vi "Process.vi"(8 "error in":errorcluster, 11 "Instrument.Lockin":refnum<class "Instrument.Lockin.lvclass">) -> (0 "error out":errorcluster, 3 "Instrument.Lockin out":refnum<class "Instrument.Lockin.lvclass">)   [LabVIEW 2019, in "Instrument.Lockin.lvlib" / "Instrument.Lockin.lvclass"]
doc: "---------------------------------------------------------------\nJKI State Machine Objects™\nhttp://jki.net/state-machine-objects/\nCopyright (C) 2005-2015, JKI <info@jki.net>\nALL RIGHTS RESERVED"
uses:
  Instrument.Lockin.lvclass
  C:/Program Files/National Instruments/LabVIEW 2019/vi.lib/JKI/JKI SMO/SMO/SMO.lvclass
  C:/Program Files/National Instruments/LabVIEW 2019/user.lib/LevyLab/Instrument Framework/Instrument/Instrument.lvclass
  Typedefs/API/Lockin.Commands.Local--Enum.ctl
  Instrument.Lockin.lvclass/Instrument.Lockin.ctl
  Typedefs/Lockin.Logging Mode--Enum.ctl
  Instrument.DAQ/Typedefs/PublicEvents--DAQ.getSweepWaveforms.ctl
  <vilib>/JKI/JKI SMO/SMO/SMO.lvclass/SMO.ctl
  Instrument.DAQ/Typedefs/Status--enum.ctl
  26abb908-d0dd-4bb2-b0ae-9417a76ac08a.vi
  58bdca10-aee7-4643-9696-ab134e43fedf.vi
  370a30f5-6ed9-43ab-971d-2debb7bc2492.vi
  5bf8e0f0-076c-483f-9499-ed5c5f42f10f.vi
  57cf7fb7-944b-4fe2-b1a2-0684563889c1.vi
  f640c324-6c77-497d-a9f4-fdf294fa3808.vi
  2ccda5d8-d2df-4877-8897-cb36dbf858a1.vi
  7ebf71aa-15a6-4da8-8ab8-2681a3011f9e.vi
  cf0dbf68-f98d-44ab-94b5-1d1e0573f492.vi
  befd05cc-8908-477d-a2f5-b8fbe5183ab0.vi
  4dcf9d6e-caf6-43ae-ab2a-813b64901b82.vi
  0479806f-3f82-4f4d-965e-31251a6a8c57.vi
  682026ae-b6e8-4d7d-90ad-286834dc1f4b.vi
  2a868a51-49ac-40d0-a5d8-0cf59a96bd77.vi
  26abb908-d0dd-4bb2-b0ae-9417a76ac08a.vi/314341ff-f36a-4754-8de1-4f8aeb5d3876.vi
  26abb908-d0dd-4bb2-b0ae-9417a76ac08a.vi/d069243e-0f6a-4917-95a4-9b44f4392aec.vi
  58bdca10-aee7-4643-9696-ab134e43fedf.vi/f87b1427-1328-4423-a40d-becc2975277f.vi
  58bdca10-aee7-4643-9696-ab134e43fedf.vi/ed747cf9-ba41-4379-ab59-768bb8ae5ff5.vi
  57cf7fb7-944b-4fe2-b1a2-0684563889c1.vi/1fd4b456-2f60-4d06-9716-df1c45004a86.vi
  57cf7fb7-944b-4fe2-b1a2-0684563889c1.vi/c11c9ad7-4649-4a85-b536-b866ca836ca1.vi
  f640c324-6c77-497d-a9f4-fdf294fa3808.vi/dbd296fc-8f34-43a8-ad34-5f6fb66ed20d.vi
  f640c324-6c77-497d-a9f4-fdf294fa3808.vi/6db23667-e41e-42f6-b96f-5bc501eef0b9.vi
  2ccda5d8-d2df-4877-8897-cb36dbf858a1.vi/344e3d59-91b1-4f61-87d6-f8dd4cdbc25b.vi
  2ccda5d8-d2df-4877-8897-cb36dbf858a1.vi/d2d6577b-fb43-4e7b-ace1-03f46b56d867.vi
  7ebf71aa-15a6-4da8-8ab8-2681a3011f9e.vi/60f027cd-f7ba-4b68-b22c-bc105befc801.vi
  7ebf71aa-15a6-4da8-8ab8-2681a3011f9e.vi/6c60f1e5-9ce0-4de3-ba4a-93b0668e9427.vi
  befd05cc-8908-477d-a2f5-b8fbe5183ab0.vi/b24fcc70-6624-4032-8476-943c5eb956bf.vi
  befd05cc-8908-477d-a2f5-b8fbe5183ab0.vi/cde51830-ddf3-45a8-9955-a1d629d46cfc.vi
  4dcf9d6e-caf6-43ae-ab2a-813b64901b82.vi/85e7a3df-5796-4879-b3a1-48313e8334c0.vi
  4dcf9d6e-caf6-43ae-ab2a-813b64901b82.vi/8e8c5bfe-5699-4deb-abb3-b8b413165a55.vi
  0479806f-3f82-4f4d-965e-31251a6a8c57.vi/af1f2937-4b31-4fa9-86ad-f8d3a4898bc2.vi
  0479806f-3f82-4f4d-965e-31251a6a8c57.vi/3be0beb5-3802-4edd-aa59-089ac39f706e.vi
  <vilib>/dlg_ctls.llb/Space Constant.vi
  <vilib>/AdvancedString/1D String Array to Delimited String.vi
  <vilib>/JKI/JKI SMO/SMO/Private/ReftoDVR--SMO.vi
  <vilib>/Utility/Data Type/Get Type Information.vi
  <vilib>/Utility/Data Type/Get Numeric Information.vi
  <userlib>/_OpenG.lib/lvdata/lvdata.llb/Unwrap VVariant__ogtk.vi
  <vilib>/JDP Science/JSONtext/Variant to JSON Text.vi
  <userlib>/LevyLab/Instrument Framework/Instrument/API/Instrument.sendMessageToProcess (string).vi
  <vilib>/JDP Science/JSONtext/LVClass Serializer/JSONtext LVClass Serializer.lvclass
  <vilib>/JKI/JKI SMO/SMO/SMO.lvclass
  <userlib>/LevyLab/Instrument Framework/Instrument Types/Lockin/Instrument.LockinAPI.lvclass
  <userlib>/LevyLab/Debug/Debug.lvlib
  Instrument.DAQ/Instrument.DAQ.lvclass
  <userlib>/LevyLab/Instrument Framework/Instrument/Instrument.lvclass
panel:
  in  "LOG":bool
  out "String":string
  # "Multichannel Lockin"
  # "For instructions on how to use the JKI State Machine Objects, examples and video tutorials, visit:\nhttp://jki.net/state-machine-objects/\n\nJKI State Machine Objects™\nhttp://jki.net/state-machine-objects/\nCopyright (C) 2005-2015, JKI <info@jki.net>\nALL RIGHTS RESERVED"
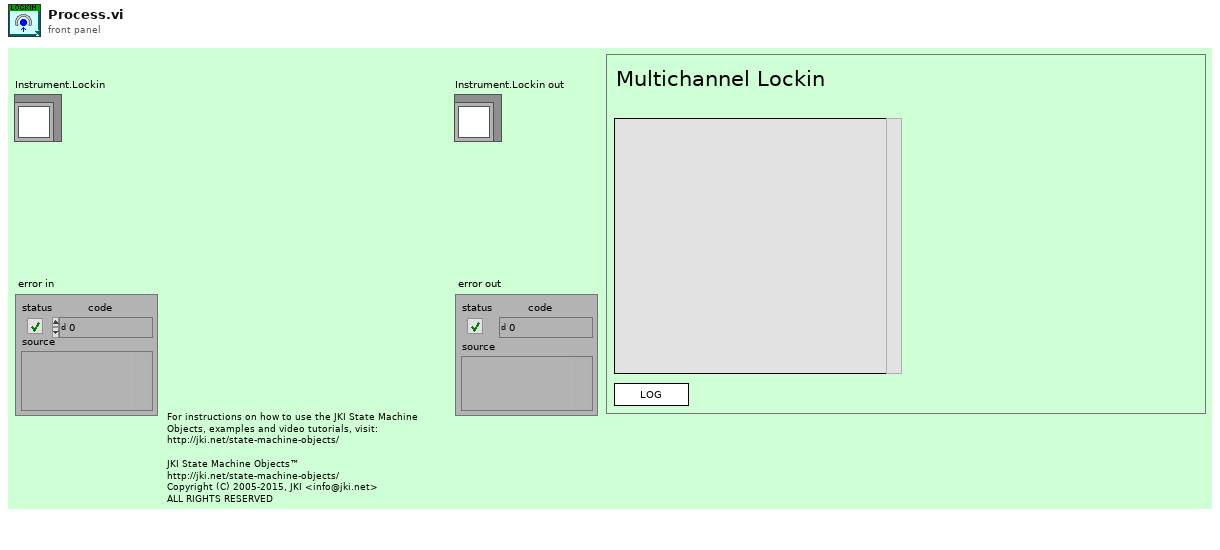
[diagram p1: front panel]
types:
  T1 = typedef "Instrument.Lockin.lvlib/Instrument.Lockin.lvclass/Lockin.Commands.Local--Enum.ctl" = enum16{"autoConfigureDAQ", "setSimulationMode", "zeroPhase", "setCalibration", "setPreFilter", "setFrequencyLink", "setAmplitudeLimit", "setDCLimit", "setDutyCycle", "setSamplingDecimationPreDSP", "setSamplingDecimationPostDSP", "setSamplingMode", "setSamplingFsMultiplier", "setSamplingFsOutput", "setSamplingRefreshRate", "setData_State", "setData_DAQ", "setData_Sampling", "setData_Waveforms", "setData_Results", "setData_SweepWaveforms", "setData_AIChannels", "setData_AOChannels", "setData_REFChannels", "setData_InputGain", "setData_OutputGain", "showUI", "setAI", "setOffset", "setOffsetMode"}
  T2 = typedef "Instrument.Lockin.lvlib/Instrument.Lockin.lvclass/Lockin.Logging Mode--Enum.ctl" = enum16{"enabled", "disabled"}
  T3 = enum32{"invalid app kind", "Development System", "Run Time System", "Student Edition", "Embedded LabVIEW", "Evaluation", "Custom"}
  T4 = enum32{"Invalid", "Standard", "Closed", "Hidden", "Minimized", "Maximized"}
  T5 = typedef "Instrument.Lockin.lvlib/Instrument.DAQ.lvclass/Status--enum.ctl" = enum16{"idle", "created", "started", "stopped", "sweeping"}
  T6 = typedef "Instrument.Lockin.lvlib/Instrument.DAQ.lvclass/PublicEvents--DAQ.getSweepWaveforms.ctl" = cluster{"AO":waveform(dbl)[], "AI":waveform(dbl)[], "X":waveform(dbl)[], "Y":waveform(dbl)[]}
  T7 = typedef "SMO.lvclass/SMOState --Enum.ctl" = enum16{"unknown", "Created", "Started", "Stopped"}
  T8 = cluster{"Core":cluster{"Current VI Reference":refnum<vi>, "Close Panel on Exit?":bool, "Last Error":cluster{"error":errorcluster, "previous state":string, "remaining states":string}, "Shutdown?":bool}, "SelfRef":refnum<class "Instrument.Lockin.lvclass">, "logConfiguration":bool, "SweepWaveformsBuffer":T6}
  T9 = typedef "Instrument.Lockin.lvlib/Instrument.DAQ.lvclass/DAQ.Configuration--Cluster--Array.ctl" = T10[]
  T10 = typedef "Instrument.Lockin.lvlib/Instrument.DAQ.lvclass/DAQ.Configuration--Cluster.ctl" = cluster{"Device":string, "Lockin.AO":string, "AO.Ch":string, "AO.Range":T11, "AO terminal config":T12, "Lockin.AI":string, "AI.Ch":string, "AI.Range":T13, "AI.Coupling":T14, "AI terminal config":T12}
  T11 = typedef "Instrument.Lockin.lvlib/Instrument.DAQ.lvclass/DAQ.Config.AO.Range--enum.ctl" = enum16{"±0.1", "±1.0", "±3.5", "±10.0", ""}
  T12 = typedef "Instrument.Lockin.lvlib/Instrument.DAQ.lvclass/DAQ.TerminalConfiguration--ring.ctl" = i32
  T13 = typedef "Instrument.Lockin.lvlib/Instrument.DAQ.lvclass/DAQ.Config.AI.Range--enum.ctl" = enum16{"±0.316", "±1.00", "±3.16", "±10.0", "±31.6", "±42.4", ""}
  T14 = typedef "Instrument.Lockin.lvlib/Instrument.DAQ.lvclass/DAQ.Config.AI.Coupling--enum.ctl" = u16
  T15 = typedef "Instrument.Lockin.lvlib/Instrument.DAQ.lvclass/DAQ.Config.AO--Cluster--Array.ctl" = cluster{"Channels":tag, "Range":T11, "terminal configuration":T12, "Type":T16}[]
  T16 = typedef "Instrument.Lockin.lvlib/Instrument.DAQ.lvclass/DAQ.Type--enum.ctl" = enum16{"None", "USB-4431", "PXI-446x"}
  T17 = typedef "Instrument.Lockin.lvlib/Instrument.DAQ.lvclass/DAQ.Config.AI--Cluster--Array.ctl" = cluster{"Channels":tag, "Coupling":T14, "Range":T13, "terminal configuration":T12, "Type":T16}[]
  T18 = typedef "Instrument.Lockin.lvlib/Instrument.DAQ.lvclass/DAQ.Sampling--Cluster.ctl" = cluster{"Sampling":T19, "sample mode":i32, "Fs Mode":T20, "Fs Multiplier":dbl, "Refresh Rate (Hz)":dbl, "Decimation.PreDSP":i32, "Decimation.PostDSP":i32, "Fs.Output":dbl}
  T19 = typedef "Instrument.Lockin.lvlib/Instrument.DAQ.lvclass/DAQ.Sampling.Sampling--Cluster.ctl" = cluster{"Fs":dbl, "#s":i32}
  T20 = typedef "Instrument.Lockin.lvlib/Instrument.DAQ.lvclass/DAQ.Sampling.Fs Mode--enum.ctl" = enum16{"Manual", "Auto Fs", "Max Fs"}
  T21 = typedef "Instrument.Lockin.lvlib/Instrument.DAQ.lvclass/AI.Channel--Cluster--Array.ctl" = T22[]
  T22 = typedef "Instrument.Lockin.lvlib/Instrument.DAQ.lvclass/AI.Channel--Cluster.ctl" = cluster{"Enable?":bool, "Channel":i32, "References":u16[], "reference index":i32}
  T23 = typedef "Instrument.Lockin.lvlib/Instrument.DAQ.lvclass/AO.Channel--Cluster--Array.ctl" = T24[]
  T24 = typedef "Instrument.Lockin.lvlib/Instrument.DAQ.lvclass/AO.Channel--Cluster.ctl" = cluster{"Enable?":bool, "Channel":i32, "Amplitude":dbl, "Offset":dbl, "Frequency":dbl, "Phase":dbl, "Function":T25, "Sweeping?":bool, "Limit AC":bool, "Limit DC?":bool, "Duty Cycle":bool}
  T25 = typedef "Instrument.Lockin.lvlib/Instrument.DAQ.lvclass/AO.Channel.Function--Enum.ctl" = enum16{"sine", "square", "triangle", "saw"}
  T26 = typedef "Instrument.Lockin.lvlib/Instrument.DAQ.lvclass/REF.Channel--Cluster--Array.ctl" = T27[]
  T27 = typedef "Instrument.Lockin.lvlib/Instrument.DAQ.lvclass/REF.Channel--Cluster.ctl" = cluster{"Enable?":bool, "Channel":i32, "Frequency":dbl, "Phase":dbl, "TC":dbl, "Roll-Off":i32}
  T28 = typedef "Instrument.Lockin.lvlib/Instrument.DAQ.lvclass/PublicEvents--DAQ.getWaveforms.ctl" = cluster{"AO":waveform(dbl)[], "AI":waveform(dbl)[], "REF_X":waveform(dbl)[], "REF_Y":waveform(dbl)[], "X":waveform(dbl)[], "Y":waveform(dbl)[]}
  T29 = typedef "Instrument.Lockin.lvlib/Instrument.DAQ.lvclass/Results--Cluster.ctl" = cluster{"Time Stamp":timestamp, "Results (Dictionary)":cluster{"key":string, "value":dbl[]}[]}
  T30 = typedef "Instrument.Lockin.lvlib/Instrument.DAQ.lvclass/DeviceInfo--Cluster.ctl" = cluster{"DeviceName":string, "DevIsSimulated":bool, "DeviceSerialNumber":string, "ProductType":string, "ProductCategory":i32, "ProductNumber":u32, "ChassisNumber":u32, "SlotNumber":u32, "ChassisName":string, "ChassisSerialNumber":string, "DevTemp":dbl, "SelfCal.LastDate/Time":string, "SelfCal.LastTemp":dbl, "calibration due?":bool}
  T31 = typedef "Instrument.Lockin.lvlib/Instrument.DAQ.lvclass/DAQ.Calibration--Cluster--Array.ctl" = T32[]
  T32 = typedef "Instrument.Lockin.lvlib/Instrument.DAQ.lvclass/DAQ.Calibration--Cluster.ctl" = cluster{"Active Device":string, "SelfCal.LastDate/Time":dbl, "SelfCal.LastTemp":dbl, "DevTemp":dbl, "calibration due?":bool}
  T33 = cluster{"Current VI Reference":refnum<vi>, "Close Panel on Exit?":bool, "Last Error":cluster{"error":errorcluster, "previous state":string, "remaining states":string}, "Shutdown?":bool}
  T34 = typedef "Debug.lvlib/Attribute.Debug.lvclass/DebugBehavior.ctl" = enum16{"Normal", "Debug"}
  T35 = typedef "SMO.lvclass/Protected Events.ctl" = cluster{"StopProcesses":refnum<user-event>, "AbortProcesses":refnum<user-event>, "Config Changed":refnum<user-event>, "Dependency":refnum<user-event>}
  T36 = typedef "SMO.lvclass/Public Events.ctl" = cluster{"Error":refnum<user-event>, "State":refnum<user-event>, "Reserve State":refnum<user-event>}
  T37 = typedef "Instrument.Lockin.lvlib/Instrument.DAQ.lvclass/PublicEvents--Cluster.ctl" = cluster{"getAIChannels":refnum<user-event>, "getAOChannels":refnum<user-event>, "getREFChannels":refnum<user-event>, "getWaveforms":refnum<user-event>, "getResults":refnum<user-event>, "getSweepWaveforms":refnum<user-event>, "getCalibration":refnum<user-event>, "getDAQState":refnum<user-event>, "getDAQconfig":refnum<user-event>, "getInputGain":refnum<user-event>, "getOutputGain":refnum<user-event>, "getInputOffset":refnum<user-event>, "getSampling":refnum<user-event>, "getSweepChannels":refnum<user-event>, "getDeviceIDN":refnum<user-event>}
  T38 = typedef "Instrument.Lockin.lvlib/Instrument.Lockin.lvclass/PrivateEvents--Cluster.ctl" = cluster{"LogInterval":refnum<user-event>, "LogConfiguration":refnum<user-event>}
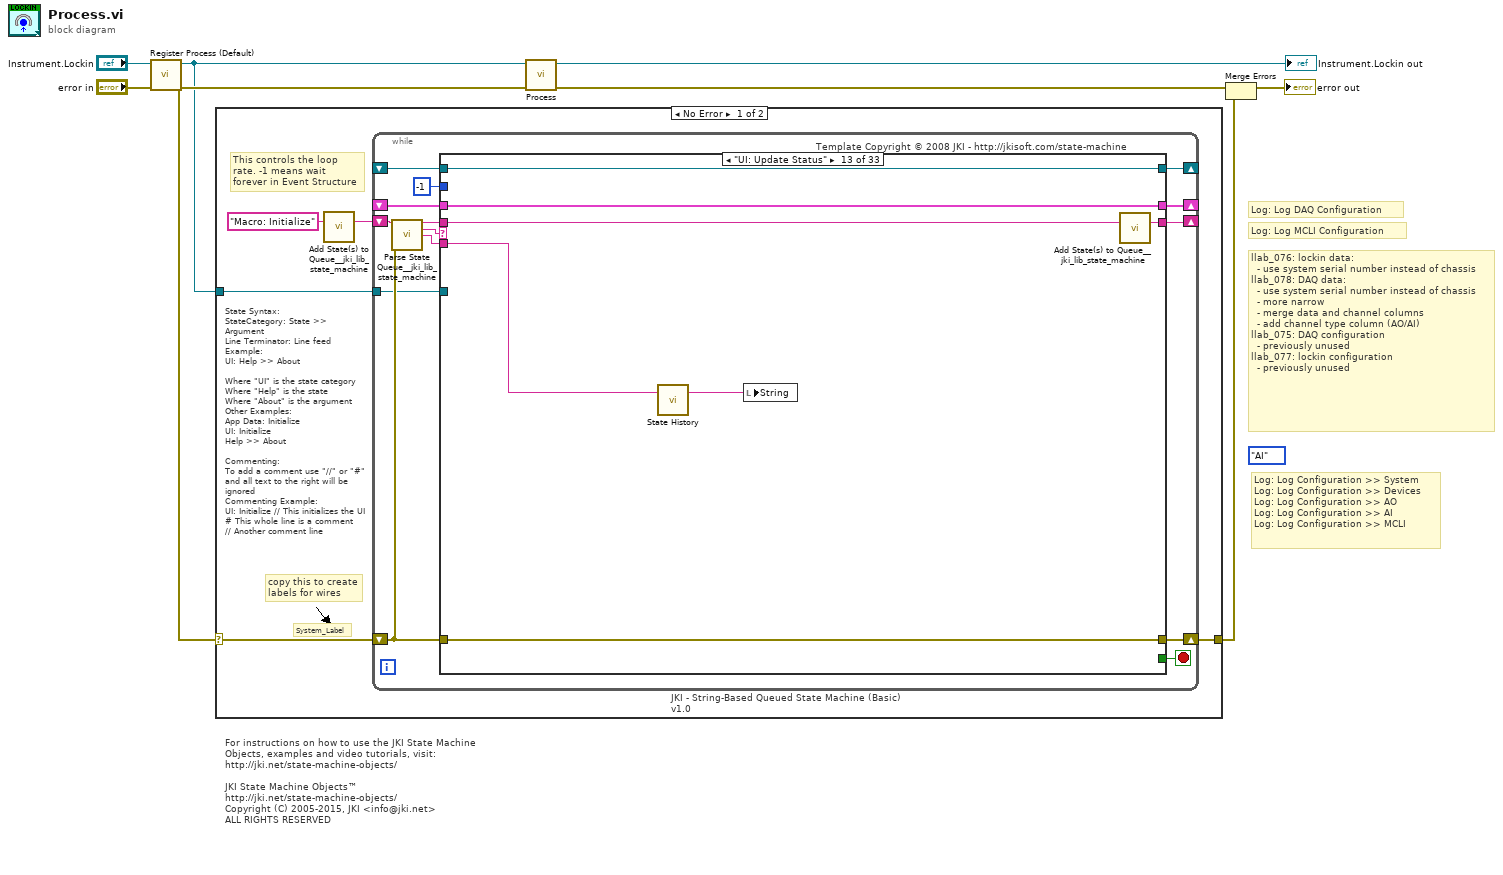
[diagram p0: block diagram]
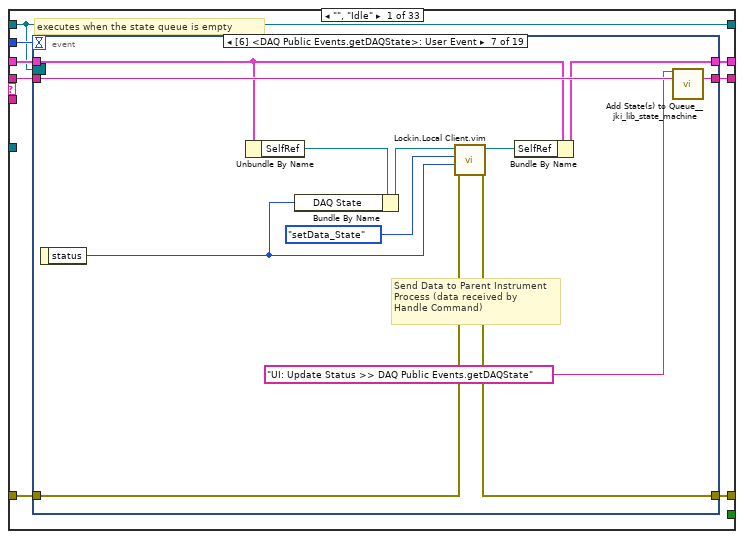
[diagram p2: hidden frame]
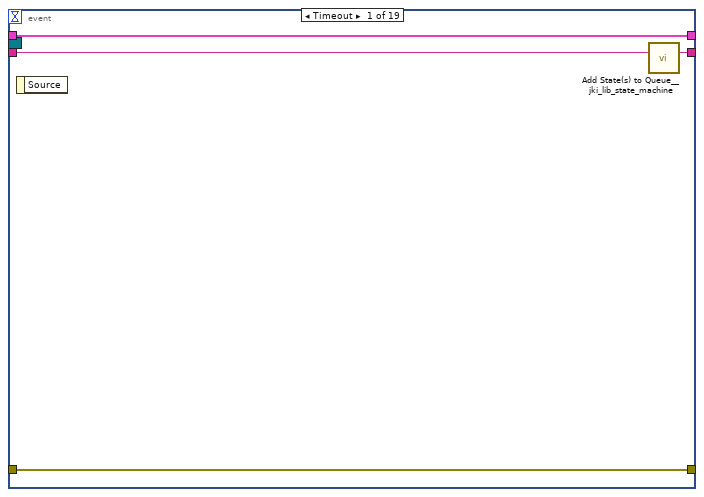
[diagram p3: hidden frame]
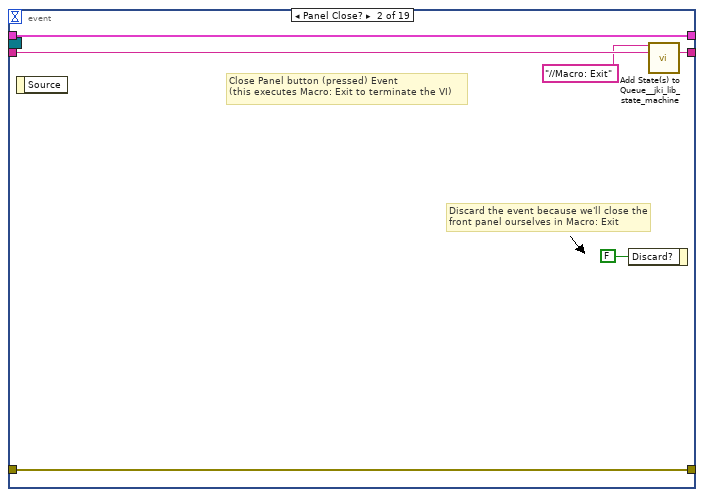
[diagram p4: hidden frame]
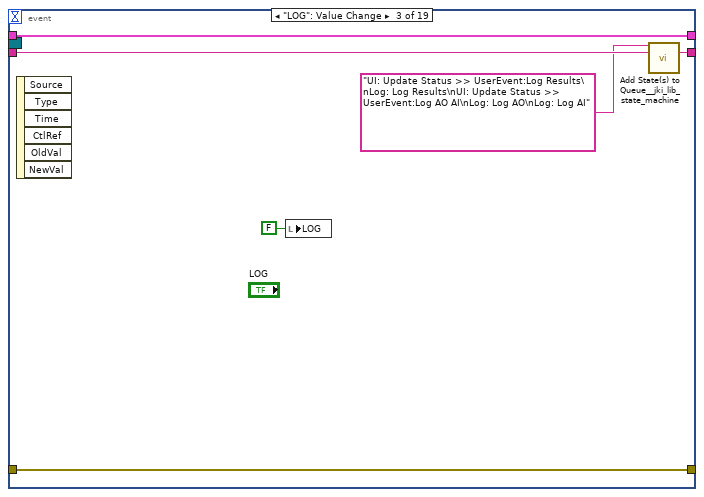
[diagram p5: hidden frame]
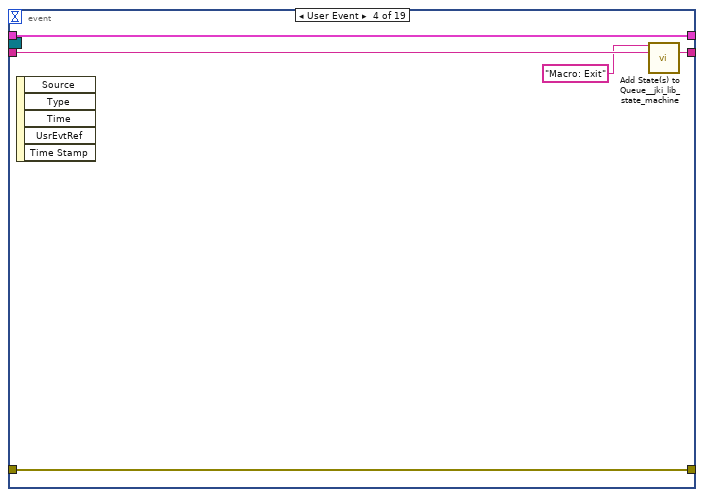
[diagram p6: hidden frame]
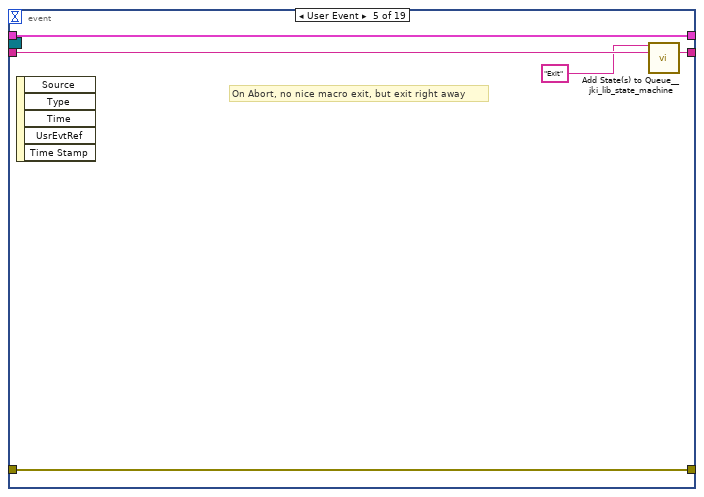
[diagram p7: hidden frame]
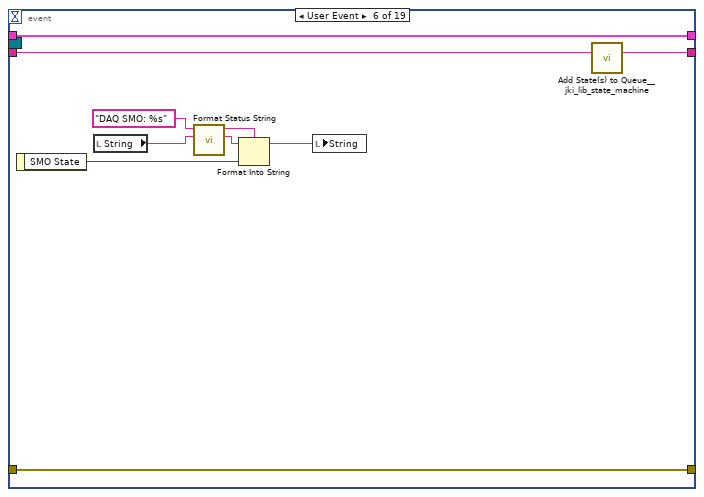
[diagram p8: hidden frame]
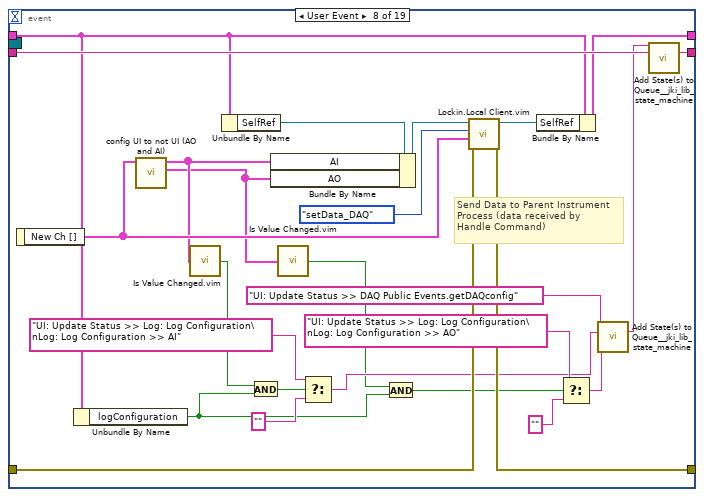
[diagram p9: hidden frame]
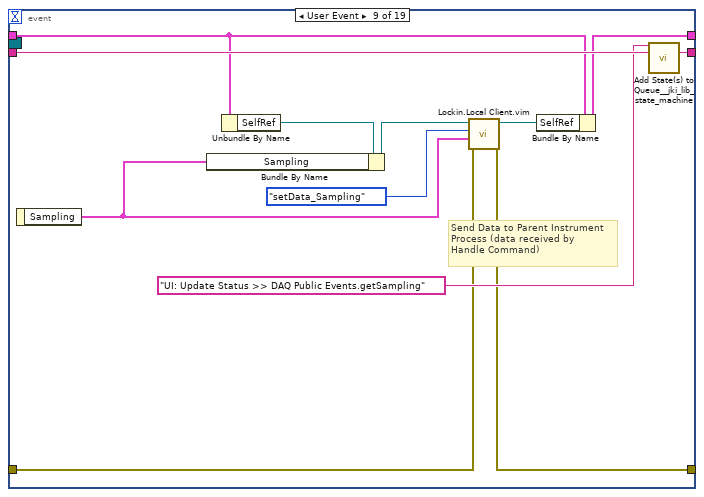
[diagram p10: hidden frame]
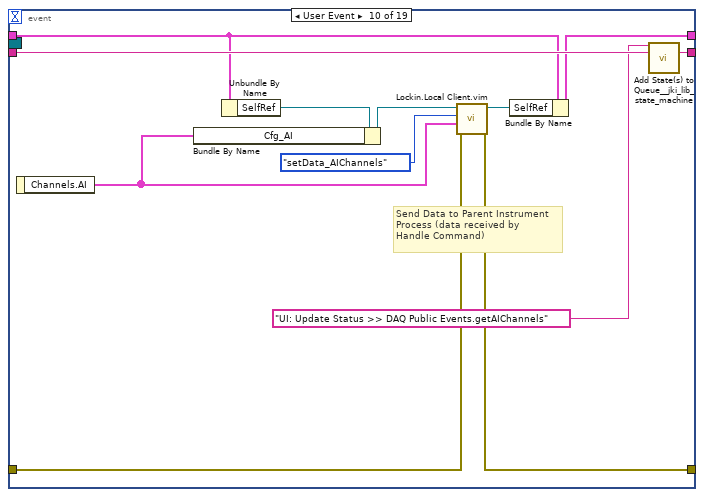
[diagram p11: hidden frame]
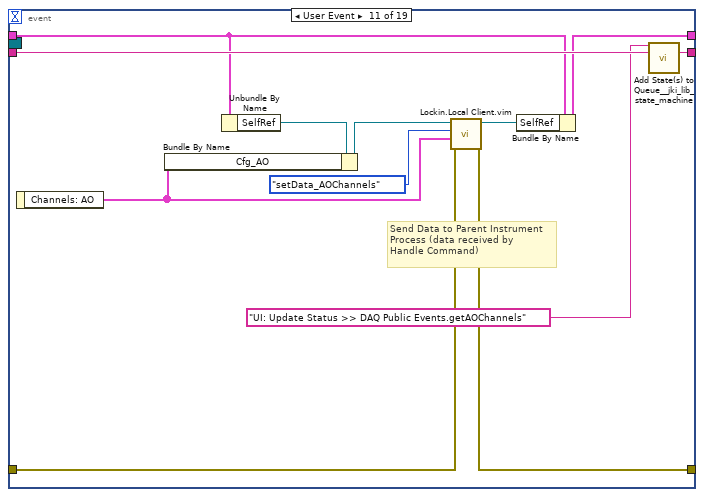
[diagram p12: hidden frame]
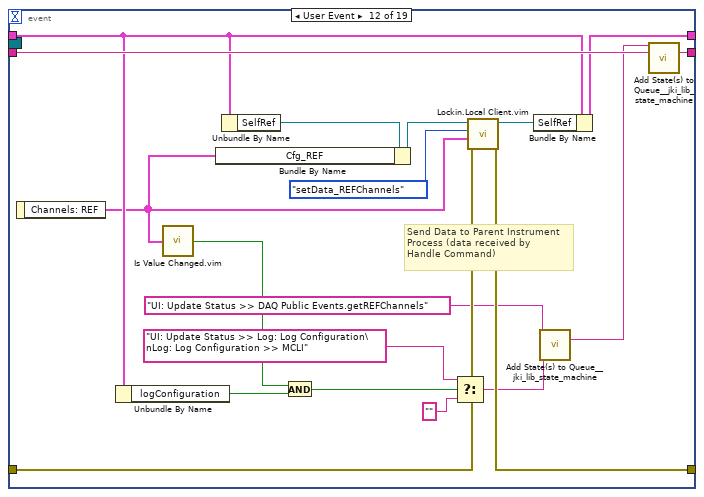
[diagram p13: hidden frame]
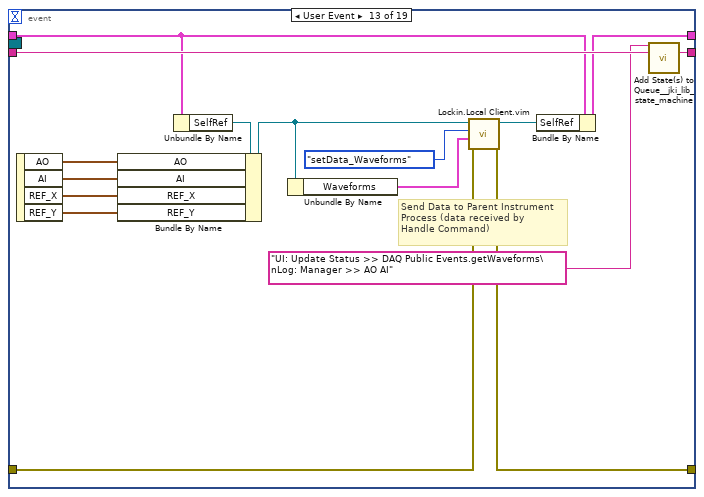
[diagram p14: hidden frame]
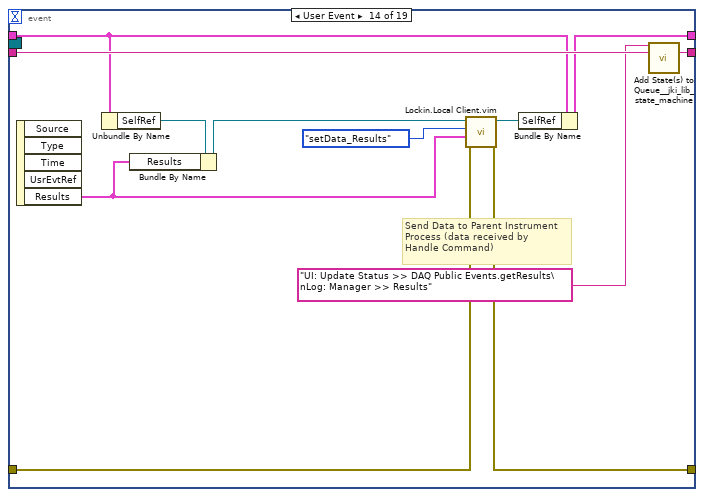
[diagram p15: hidden frame]
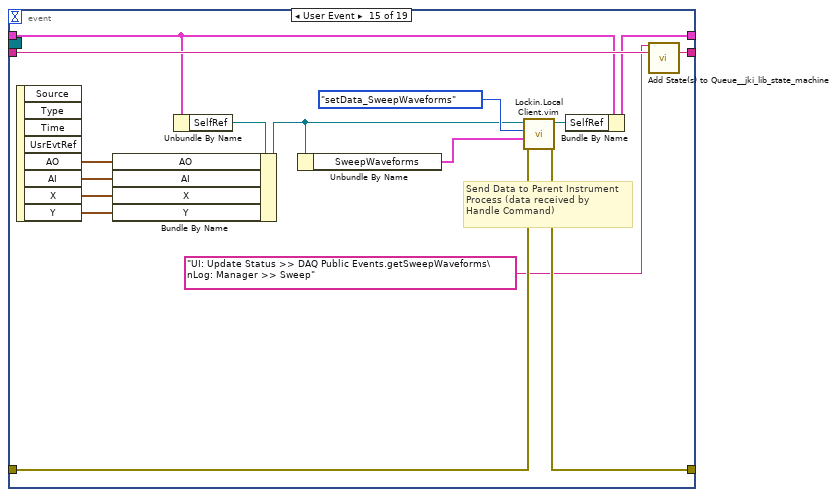
[diagram p16: hidden frame]
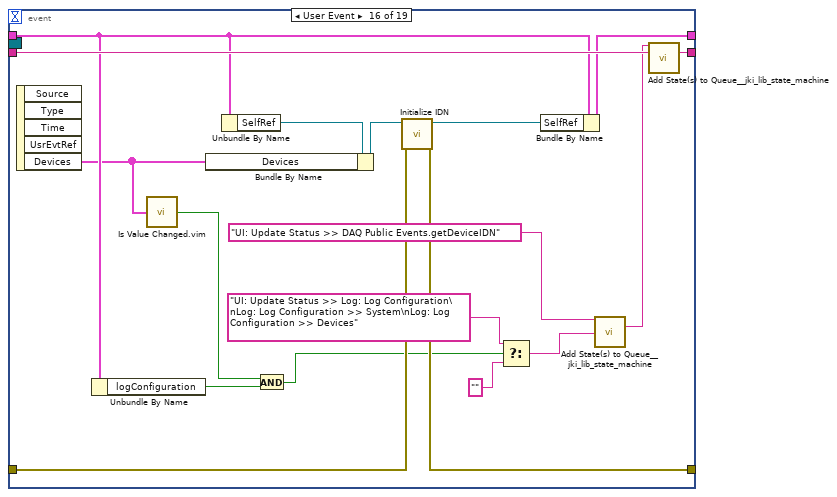
[diagram p17: hidden frame]
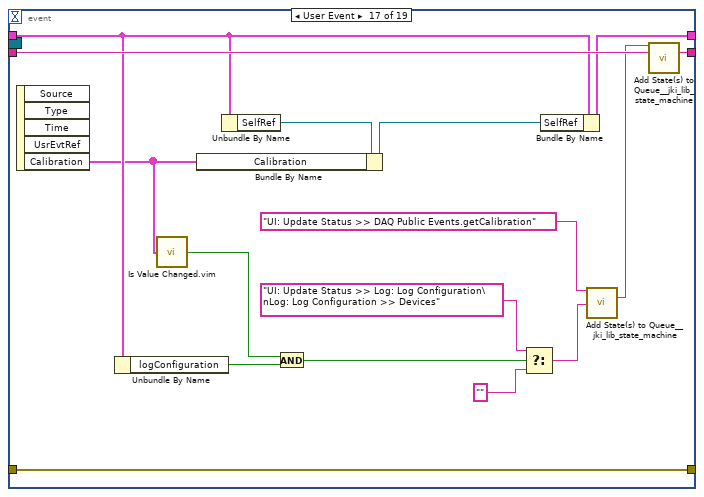
[diagram p18: hidden frame]
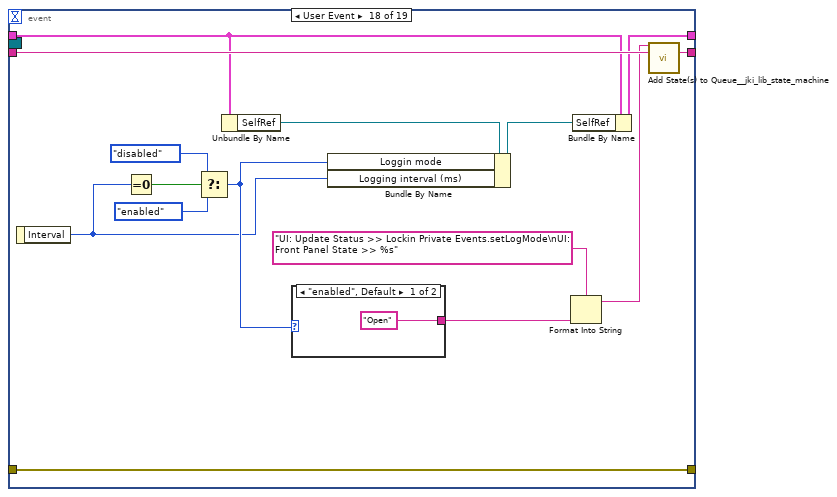
[diagram p19: hidden frame]
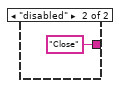
[diagram p20: hidden frame]
diagram:
  (unwired) enum16{"System", "Devices", "AO", "AI", "MCLI"}."AI" ("Enum")
  # "Log: Log Configuration >> System\nLog: Log Configuration >> Devices\nLog: Log Configuration >> AO\nLog: Log Configuration >> AI\nLog: Log Configuration >> MCLI"
  # "Log: Log DAQ Configuration"
  # "Log: Log MCLI Configuration"
  # "llab_076: lockin data:\n  - use system serial number instead of chassis\nllab_078: DAQ data:\n  - use system serial number instead of chassis\n  - more narrow\n  - merge data and channel columns\n  - add channel type column (AO/AI)\nllab_075: DAQ configuration\n  - previously unused\nllab_077: lockin configuration\n  - previously unused"
  # "For instructions on how to use the JKI State Machine Objects, examples and video tutorials, visit:\nhttp://jki.net/state-machine-objects/\n\nJKI State Machine Objects™\nhttp://jki.net/state-machine-objects/\nCopyright (C) 2005-2015, JKI <info@jki.net>\nALL RIGHTS RESERVED"
  n1 = call <vilib>:"Register Process (Default).vi"("error in (no error)"="error in", "SMO"="Instrument.Lockin") -> ("error out"=w5:errorcluster, "SelfRef"=w4:refnum<class "Instrument.Lockin.lvclass">)  [unwired: 8 in]
  n2 = case shown="No Error" w5 {
    selector: w5 -> [w10 w635]
    tunnel: w4 -> [w11 _]
    tunnel: [w9 w635] -> w1
    frame No Error {
      # "State Syntax:\nStateCategory: State >> Argument\nLine Terminator: Line feed\nExample:\nUI: Help >> About\n\nWhere \"UI\" is the state category\nWhere \"Help\" is the state\nWhere \"About\" is the argument\nOther Examples:\nApp Data: Initialize\nUI: Initialize\nHelp >> About\n\nCommenting:\nTo add a comment use \"//\" or \"#\" and all text to the right will be ignored\nCommenting Example:\nUI: Initialize // This initializes the UI\n# This whole line is a comment\n// Another comment line"
      # "copy this to create labels for wires"
      # "This controls the loop rate. -1 means wait forever in Event Structure"
      # "System_Label"
      n3 = call <vilib>:"Add State(s) to Queue__jki_lib_state_machine.vi"("State(s) in (\"\")"="Macro: Initialize") -> ("States Out"=w13:string)  [unwired: 14 in]
      n4 = while "JKI - String-Based Queued State Machine (Basic) v1.0" {
        shift-right: [w20] -> _
        shift-left: _ -> [w19]
        shift-right: [w23] -> w9
        shift-left: w10 -> [w17]
        shift-right: [w22] -> _
        shift-left: w13 -> [w24]
        tunnel: w11 -> [w16]
        shift-right: [w15] -> _
        shift-left: _ -> [w14]
        stop <- w21 stop-if-true
        # "Template Copyright © 2008 JKI - http://jkisoft.com/state-machine"
        n5 = call <vilib>:"Parse State Queue__jki_lib_state_machine.vi"("State Queue"=w24, "Error In (no error)"=w17) -> ("Remaining States"=w26:string, "Current State"=w27:string, "Arguments"=w25:string)  [unwired: 11 in]
        n6 = case shown="\"UI: Update Status\"" w27 {
          selector: w27 -> [_ _ w274 _ _ _ _ _ _ _ _ _ _ _ _ _ _ _ _ _ _ _ _ _ _ _ _ _ _ _ _ _ _]
          tunnel: w26 -> [w35 w272 w278 w297 w299 w316 w321 w333 w340 w359 w364 w372 w379 w388 w395 w411 w443 w452 w464 w483 w504 w509 w520 w525 w542 w548 w553 w564 w601 w608 w615 w622 w634]
          tunnel: w25 -> [_ _ _ _ _ _ _ _ _ _ _ _ w373 w380 w389 w405 _ _ _ _ _ _ _ _ _ _ _ w554 w592 _ _ _ _]
          tunnel: w19 -> [w33 w269 w276 w288 w306 w312 w318 _ w335 w349 w361 w370 w376 w385 w393 w407 w440 w444 w453 w472 w489 w506 w517 w522 w536 w546 w549 w560 w598 w605 w612 w619 w626]
          tunnel: [w32 w270 w280 w294 errorcluster {"status"=FALSE, "code"=0, "source"=""} ("No error") w311 w319 w329 w336 w357 w362 w367 w377 w386 w390 w408 w441 w446 w462 w470 w502 w507 w511 w523 w538 w544 w550 w561 w596 w604 w611 w616 w629] -> w23
          tunnel: w17 -> [w31 w270 w279 w294 w308 _ w319 w329 w337 w357 w362 w366 w377 w386 w391 w409 w441 w446 w462 w469 w502 w507 w512 w523 w534 w544 w550 w561 w595 w603 w609 w617 w630]
          tunnel: [w34 w271 w277 w296 w304 w315 w320 w332 w339 w358 w363 w371 w378 w387 w394 w410 w442 w451 w463 w482 w503 w508 w519 w524 w541 w547 w552 w563 w600 w607 w614 w621 w633] -> w22
          tunnel: [_ _ _ _ _ TRUE _ _ _ _ _ _ _ _ _ _ _ _ _ _ _ _ _ _ _ _ _ _ _ _ _ _ _] -> w21
          tunnel: [w30 w269 w276 w295 w305 w312 w318 w331 w335 w350 w361 w370 w376 w385 w393 w407 w440 w444 w454 w473 w490 w506 w517 w522 w536 w546 w549 w560 w598 w605 w612 w619 w627] -> w20
          tunnel: -1 ("Timeout") -> [w29 _ _ _ _ _ _ _ _ _ _ _ _ _ _ _ _ _ _ _ _ _ _ _ _ _ _ _ _ _ _ _ _]
          tunnel: w16 -> [_ _ _ _ _ _ _ w326 _ _ _ _ _ _ _ _ _ _ _ _ _ _ _ _ _ _ _ _ _ _ _ _ _]
          tunnel: [w28 w268 w273 w285 w310 w313 w317 w330 w334 w356 w360 w369 w375 w384 w392 w404 w439 w450 w461 w481 w496 w505 w518 w521 w540 w545 w551 w562 w599 w606 w613 w620 w632] -> w15
          tunnel: w14 -> [w28 w268 w273 w285 w310 w313 w317 w330 w334 w356 w360 w369 w375 w384 w392 w404 w439 w450 w461 w481 w496 w505 w518 w521 _ w545 w551 w562 w599 w606 w613 w620 w632]
          frame "", "Idle" {
            # "executes when the state queue is empty"
            n7 = event shown="[6] <DAQ Public Events.getDAQState>: User Event" {
              selector: w28 -> [_ _ _ _ _ _ _ _ _ _ _ _ _ _ _ _ _ _ _]
              dyn-events: _ -> [_ _ _ _ _ _ _ _ _ _ _ _ _ _ _ _ _ _ _]
              timeout: w29 -> [_ _ _ _ _ _ _ _ _ _ _ _ _ _ _ _ _ _ _]
              tunnel: w35 -> [w39 w45 w51 w56 w61 w69 w83 w109 w121 w133 w145 w164 w180 w192 w208 w226 w242 w257 w267]
              tunnel: [w38 w44 w50 w55 w60 w70 w82 w108 w120 w132 w144 w163 w179 w191 w207 w225 w241 w256 w266] -> w34
              tunnel: w33 -> [w36 w42 w48 w53 w58 w68 w80 w94 w118 w130 w142 w151 w177 w189 w205 w213 w233 w254 w264]
              tunnel: [w37 w43 w49 w54 w59 w67 w77 w102 w112 w127 w136 w157 w168 w187 w197 w220 w238 w252 w263] -> w32
              tunnel: w31 -> [w37 w43 w49 w54 w59 w67 w74 w101 w111 w126 w135 w156 w167 w186 w196 w219 w238 w252 w263]
              tunnel: [w36 w42 w48 w53 w58 w68 w81 w107 w119 w131 w143 w162 w178 w190 w206 w224 w240 w255 w265] -> w30
              event Timeout {
                n8 = event-data() -> ()  [unwired: 1 in, 1 out]
                n9 = call <vilib>:"Add State(s) to Queue__jki_lib_state_machine.vi"("State(s) in (\"\")"=w39) -> ("States Out"=w38:string)  [unwired: 14 in]
              }
              event Panel Close? {
                # "Discard the event because we'll close the front panel ourselves in Macro: Exit"
                # "Close Panel button (pressed) Event\n(this executes Macro: Exit to terminate the VI)"
                n10 = event-data() -> ()  [unwired: 1 in, 1 out]
                n11 = event-data("Discard?"=FALSE) -> ()  [unwired: 1 in, 1 out]
                n12 = call <vilib>:"Add State(s) to Queue__jki_lib_state_machine.vi"("State(s) in Front (\"\")"="//Macro: Exit", "State(s) in (\"\")"=w45) -> ("States Out"=w44:string)  [unwired: 13 in]
              }
              event "LOG": Value Change {
                n13 = event-data() -> ()  [unwired: 1 in, 6 out]
                n14 = local write "LOG"(FALSE ("LOG")) -> ()
                n15 = call <vilib>:"Add State(s) to Queue__jki_lib_state_machine.vi"("State(s) in Front (\"\")"="UI: Update Status >> UserEvent:Log Results\nLog: Log Results\nUI: Update Status >> UserEvent:Log AO AI\nLog: Log AO\nLog: Log AI", "State(s) in (\"\")"=w51) -> ("States Out"=w50:string)  [unwired: 13 in]
              }
              event User Event {
                n16 = event-data() -> ()  [unwired: 1 in, 5 out]
                n17 = call <vilib>:"Add State(s) to Queue__jki_lib_state_machine.vi"("State(s) in Front (\"\")"="Macro: Exit", "State(s) in (\"\")"=w56) -> ("States Out"=w55:string)  [unwired: 13 in]
              }
              event User Event {
                # "On Abort, no nice macro exit, but exit right away"
                n18 = event-data() -> ()  [unwired: 1 in, 5 out]
                n19 = call <vilib>:"Add State(s) to Queue__jki_lib_state_machine.vi"("State(s) in Front (\"\")"="Exit", "State(s) in (\"\")"=w61) -> ("States Out"=w60:string)  [unwired: 13 in]
              }
              event User Event {
                n20 = event-data() -> ("SMO State"=w71:T7)  [unwired: 1 in]
                n21 = local read "String"() -> (w64:string)
                n22 = call "Format Status String.vi"("initial string"=w64, "format string"="DAQ SMO: %s") -> ("initial string out"=w63:string, "format string out"=w62:string)  [unwired: 8 in]
                n23 = Format Into String(format string=w62, initial string=w63, w71) -> (resulting string=w66:string)  [unwired: 1 in, 1 out]
                n24 = local write "String"(w66) -> ()
                n25 = call <vilib>:"Add State(s) to Queue__jki_lib_state_machine.vi"("State(s) in (\"\")"=w69) -> ("States Out"=w70:string)  [unwired: 14 in]
              }
              event User Event {
                # "Send Data to Parent Instrument\nProcess (data received by\nHandle Command)"
                n26 = event-data() -> ("status"=w72:T5)  [unwired: 1 in]
                n27 = Unbundle By Name(w80) -> ("SelfRef"=w76:refnum<class "Instrument.Lockin.lvclass">)
                n28 = Bundle By Name(cluster=w76, "DAQ State"=w72) -> (w75:refnum<class "Instrument.Lockin.lvclass">)
                n29 = call "Lockin.Local Client.vim"("error in (no error)"=w74, "Data"=w72, "Command"=Lockin.Commands.Local--Enum."setData_State" ("Enum"), "Instrument.Lockin in"=w75) -> ("error out"=w77:errorcluster, "Instrument.Lockin out"=w78:refnum<class "Instrument.Lockin.lvclass">)  [unwired: 6 in]
                n30 = Bundle By Name(cluster=w80, "SelfRef"=w78) -> (w81:T8)
                n31 = call <vilib>:"Add State(s) to Queue__jki_lib_state_machine.vi"("State(s) in Front (\"\")"="UI: Update Status >> DAQ Public Events.getDAQState" ("State(s) in Front (\"\")"), "State(s) in (\"\")"=w83) -> ("States Out"=w82:string)  [unwired: 13 in]
              }
              event User Event {
                # "Send Data to Parent Instrument\nProcess (data received by\nHandle Command)"
                n32 = event-data() -> ("New Ch []"=w103:T9)  [unwired: 1 in]
                n33 = Unbundle By Name(w94) -> ("logConfiguration"=w86:bool)
                n34 = call "config UI to not UI (AO and AI).vi"("New Ch []"=w103) -> ("AO Config"=w89:T15, "AI Config"=w93:T17)  [unwired: 9 in]
                n35 = call "Is Value Changed.vim"("value"=w93) -> ("changed or first call?"=w88:bool)
                n36 = Unbundle By Name(w94) -> ("SelfRef"=w106:refnum<class "Instrument.Lockin.lvclass">)
                n37 = And(x=w88, y=w86) -> (x .and. y?=w92:bool)
                n38 = Bundle By Name(cluster=w106, "AI"=w93, "AO"=w89) -> (w105:refnum<class "Instrument.Lockin.lvclass">)
                n39 = call "Is Value Changed.vim"("value"=w89) -> ("changed or first call?"=w85:bool)
                n40 = Select(t="UI: Update Status >> Log: Log Configuration\nLog: Log Configuration >> AI" ("State(s) in Front (\"\")"), s=w92, f="") -> (s? t:f=w87:string)
                n41 = And(x=w85, y=w86) -> (x .and. y?=w84:bool)
                n42 = call "Lockin.Local Client.vim"("error in (no error)"=w101, "Data"=w103, "Command"=Lockin.Commands.Local--Enum."setData_DAQ" ("Enum"), "Instrument.Lockin in"=w105) -> ("error out"=w102:errorcluster, "Instrument.Lockin out"=w104:refnum<class "Instrument.Lockin.lvclass">)  [unwired: 6 in]
                n43 = Bundle By Name(cluster=w94, "SelfRef"=w104) -> (w107:T8)
                n44 = Select(t="UI: Update Status >> Log: Log Configuration\nLog: Log Configuration >> AO" ("State(s) in Front (\"\")"), s=w84, f="") -> (s? t:f=w97:string)
                n45 = call <vilib>:"Add State(s) to Queue__jki_lib_state_machine.vi"("State(s) in Front (\"\")"="UI: Update Status >> DAQ Public Events.getDAQconfig" ("State(s) in Front (\"\")"), "State(s) in (\"\")"=w87, "State(s) at Back (\"\")"=w97) -> ("States Out"=w95:string)  [unwired: 12 in]
                n46 = call <vilib>:"Add State(s) to Queue__jki_lib_state_machine.vi"("State(s) in Front (\"\")"=w95, "State(s) in (\"\")"=w109) -> ("States Out"=w108:string)  [unwired: 13 in]
              }
              event User Event {
                # "Send Data to Parent Instrument\nProcess (data received by\nHandle Command)"
                n47 = event-data() -> ("Sampling"=w110:T18)  [unwired: 1 in]
                n48 = Unbundle By Name(w118) -> ("SelfRef"=w117:refnum<class "Instrument.Lockin.lvclass">)
                n49 = Bundle By Name(cluster=w117, "Sampling"=w110) -> (w114:refnum<class "Instrument.Lockin.lvclass">)
                n50 = call "Lockin.Local Client.vim"("error in (no error)"=w111, "Data"=w110, "Command"=Lockin.Commands.Local--Enum."setData_Sampling" ("Enum"), "Instrument.Lockin in"=w114) -> ("error out"=w112:errorcluster, "Instrument.Lockin out"=w113:refnum<class "Instrument.Lockin.lvclass">)  [unwired: 6 in]
                n51 = Bundle By Name(cluster=w118, "SelfRef"=w113) -> (w119:T8)
                n52 = call <vilib>:"Add State(s) to Queue__jki_lib_state_machine.vi"("State(s) in Front (\"\")"="UI: Update Status >> DAQ Public Events.getSampling" ("State(s) in Front (\"\")"), "State(s) in (\"\")"=w121) -> ("States Out"=w120:string)  [unwired: 13 in]
              }
              event User Event {
                # "Send Data to Parent Instrument\nProcess (data received by\nHandle Command)"
                n53 = event-data() -> ("Channels.AI"=w122:T21)  [unwired: 1 in]
                n54 = Unbundle By Name(w130) -> ("SelfRef"=w129:refnum<class "Instrument.Lockin.lvclass">)
                n55 = Bundle By Name(cluster=w129, "Cfg_AI"=w122) -> (w125:refnum<class "Instrument.Lockin.lvclass">)
                n56 = call "Lockin.Local Client.vim"("error in (no error)"=w126, "Data"=w122, "Command"=Lockin.Commands.Local--Enum."setData_AIChannels" ("Enum"), "Instrument.Lockin in"=w125) -> ("error out"=w127:errorcluster, "Instrument.Lockin out"=w124:refnum<class "Instrument.Lockin.lvclass">)  [unwired: 6 in]
                n57 = Bundle By Name(cluster=w130, "SelfRef"=w124) -> (w131:T8)
                n58 = call <vilib>:"Add State(s) to Queue__jki_lib_state_machine.vi"("State(s) in Front (\"\")"="UI: Update Status >> DAQ Public Events.getAIChannels" ("State(s) in Front (\"\")"), "State(s) in (\"\")"=w133) -> ("States Out"=w132:string)  [unwired: 13 in]
              }
              event User Event {
                # "Send Data to Parent Instrument\nProcess (data received by\nHandle Command)"
                n59 = event-data() -> ("Channels: AO"=w138:T23)  [unwired: 1 in]
                n60 = Unbundle By Name(w142) -> ("SelfRef"=w141:refnum<class "Instrument.Lockin.lvclass">)
                n61 = Bundle By Name(cluster=w141, "Cfg_AO"=w138) -> (w137:refnum<class "Instrument.Lockin.lvclass">)
                n62 = call "Lockin.Local Client.vim"("error in (no error)"=w135, "Data"=w138, "Command"=Lockin.Commands.Local--Enum."setData_AOChannels" ("Enum"), "Instrument.Lockin in"=w137) -> ("error out"=w136:errorcluster, "Instrument.Lockin out"=w134:refnum<class "Instrument.Lockin.lvclass">)  [unwired: 6 in]
                n63 = Bundle By Name(cluster=w142, "SelfRef"=w134) -> (w143:T8)
                n64 = call <vilib>:"Add State(s) to Queue__jki_lib_state_machine.vi"("State(s) in Front (\"\")"="UI: Update Status >> DAQ Public Events.getAOChannels" ("State(s) in Front (\"\")"), "State(s) in (\"\")"=w145) -> ("States Out"=w144:string)  [unwired: 13 in]
              }
              event User Event {
                # "Send Data to Parent Instrument\nProcess (data received by\nHandle Command)"
                n65 = event-data() -> ("Channels: REF"=w146:T26)  [unwired: 1 in]
                n66 = Unbundle By Name(w151) -> ("logConfiguration"=w149:bool)
                n67 = call "Is Value Changed.vim"("value"=w146) -> ("changed or first call?"=w147:bool)
                n68 = Unbundle By Name(w151) -> ("SelfRef"=w161:refnum<class "Instrument.Lockin.lvclass">)
                n69 = Bundle By Name(cluster=w161, "Cfg_REF"=w146) -> (w159:refnum<class "Instrument.Lockin.lvclass">)
                n70 = And(x=w147, y=w149) -> (x .and. y?=w148:bool)
                n71 = Select(t="UI: Update Status >> Log: Log Configuration\nLog: Log Configuration >> MCLI" ("State(s) in Front (\"\")"), s=w148, f="") -> (s? t:f=w153:string)
                n72 = call "Lockin.Local Client.vim"("error in (no error)"=w156, "Data"=w146, "Command"=Lockin.Commands.Local--Enum."setData_REFChannels" ("Enum"), "Instrument.Lockin in"=w159) -> ("error out"=w157:errorcluster, "Instrument.Lockin out"=w158:refnum<class "Instrument.Lockin.lvclass">)  [unwired: 6 in]
                n73 = Bundle By Name(cluster=w151, "SelfRef"=w158) -> (w162:T8)
                n74 = call <vilib>:"Add State(s) to Queue__jki_lib_state_machine.vi"("State(s) in Front (\"\")"="UI: Update Status >> DAQ Public Events.getREFChannels" ("State(s) in Front (\"\")"), "State(s) at Back (\"\")"=w153) -> ("States Out"=w152:string)  [unwired: 13 in]
                n75 = call <vilib>:"Add State(s) to Queue__jki_lib_state_machine.vi"("State(s) in Front (\"\")"=w152, "State(s) in (\"\")"=w164) -> ("States Out"=w163:string)  [unwired: 13 in]
              }
              event User Event {
                # "Send Data to Parent Instrument\nProcess (data received by\nHandle Command)"
                n76 = event-data() -> ("AO"=w175:waveform(dbl)[], "AI"=w174:waveform(dbl)[], "REF_X"=w173:waveform(dbl)[], "REF_Y"=w172:waveform(dbl)[])  [unwired: 1 in]
                n77 = Unbundle By Name(w177) -> ("SelfRef"=w176:refnum<class "Instrument.Lockin.lvclass">)
                n78 = Bundle By Name(cluster=w176, "AO"=w175, "AI"=w174, "REF_X"=w173, "REF_Y"=w172) -> (w170:refnum<class "Instrument.Lockin.lvclass">)
                n79 = Unbundle By Name(w170) -> ("Waveforms"=w169:T28)
                n80 = call "Lockin.Local Client.vim"("error in (no error)"=w167, "Data"=w169, "Command"=Lockin.Commands.Local--Enum."setData_Waveforms" ("Enum"), "Instrument.Lockin in"=w170) -> ("error out"=w168:errorcluster, "Instrument.Lockin out"=w171:refnum<class "Instrument.Lockin.lvclass">)  [unwired: 6 in]
                n81 = Bundle By Name(cluster=w177, "SelfRef"=w171) -> (w178:T8)
                n82 = call <vilib>:"Add State(s) to Queue__jki_lib_state_machine.vi"("State(s) in Front (\"\")"="UI: Update Status >> DAQ Public Events.getWaveforms\nLog: Manager >> AO AI" ("State(s) in Front (\"\")"), "State(s) in (\"\")"=w180) -> ("States Out"=w179:string)  [unwired: 13 in]
              }
              event User Event {
                # "Send Data to Parent Instrument\nProcess (data received by\nHandle Command)"
                n83 = event-data() -> ("Results"=w184:T29)  [unwired: 1 in, 4 out]
                n84 = Unbundle By Name(w189) -> ("SelfRef"=w183:refnum<class "Instrument.Lockin.lvclass">)
                n85 = Bundle By Name(cluster=w183, "Results"=w184) -> (w182:refnum<class "Instrument.Lockin.lvclass">)
                n86 = call "Lockin.Local Client.vim"("error in (no error)"=w186, "Data"=w184, "Command"=Lockin.Commands.Local--Enum."setData_Results" ("Enum"), "Instrument.Lockin in"=w182) -> ("error out"=w187:errorcluster, "Instrument.Lockin out"=w185:refnum<class "Instrument.Lockin.lvclass">)  [unwired: 6 in]
                n87 = Bundle By Name(cluster=w189, "SelfRef"=w185) -> (w190:T8)
                n88 = call <vilib>:"Add State(s) to Queue__jki_lib_state_machine.vi"("State(s) in Front (\"\")"="UI: Update Status >> DAQ Public Events.getResults\nLog: Manager >> Results" ("State(s) in Front (\"\")"), "State(s) in (\"\")"=w192) -> ("States Out"=w191:string)  [unwired: 13 in]
              }
              event User Event {
                # "Send Data to Parent Instrument\nProcess (data received by\nHandle Command)"
                n89 = event-data() -> ("AO"=w203:waveform(dbl)[], "AI"=w202:waveform(dbl)[], "X"=w201:waveform(dbl)[], "Y"=w200:waveform(dbl)[])  [unwired: 1 in, 4 out]
                n90 = Unbundle By Name(w205) -> ("SelfRef"=w204:refnum<class "Instrument.Lockin.lvclass">)
                n91 = Bundle By Name(cluster=w204, "AO"=w203, "AI"=w202, "X"=w201, "Y"=w200) -> (w195:refnum<class "Instrument.Lockin.lvclass">)
                n92 = Unbundle By Name(w195) -> ("SweepWaveforms"=w194:T6)
                n93 = call "Lockin.Local Client.vim"("error in (no error)"=w196, "Data"=w194, "Command"=Lockin.Commands.Local--Enum."setData_SweepWaveforms" ("Enum"), "Instrument.Lockin in"=w195) -> ("error out"=w197:errorcluster, "Instrument.Lockin out"=w198:refnum<class "Instrument.Lockin.lvclass">)  [unwired: 6 in]
                n94 = Bundle By Name(cluster=w205, "SelfRef"=w198) -> (w206:T8)
                n95 = call <vilib>:"Add State(s) to Queue__jki_lib_state_machine.vi"("State(s) in Front (\"\")"="UI: Update Status >> DAQ Public Events.getSweepWaveforms\nLog: Manager >> Sweep" ("State(s) in Front (\"\")"), "State(s) in (\"\")"=w208) -> ("States Out"=w207:string)  [unwired: 13 in]
              }
              event User Event {
                n96 = event-data() -> ("Devices"=w212:T30[])  [unwired: 1 in, 4 out]
                n97 = Unbundle By Name(w213) -> ("logConfiguration"=w211:bool)
                n98 = call "Is Value Changed.vim"("value"=w212) -> ("changed or first call?"=w209:bool)
                n99 = Unbundle By Name(w213) -> ("SelfRef"=w223:refnum<class "Instrument.Lockin.lvclass">)
                n100 = Bundle By Name(cluster=w223, "Devices"=w212) -> (w222:refnum<class "Instrument.Lockin.lvclass">)
                n101 = And(x=w209, y=w211) -> (x .and. y?=w210:bool)
                n102 = call <userlib>:"Initialize IDN.vi"("error in (no error)"=w219, "Instrument in"=w222) -> ("error out"=w220:errorcluster, "Instrument out"=w221:refnum<class "Instrument.Lockin.lvclass">)  [unwired: 8 in]
                n103 = Select(t="UI: Update Status >> Log: Log Configuration\nLog: Log Configuration >> System\nLog: Log Configuration >> Devices" ("State(s) in Front (\"\")"), s=w210, f="") -> (s? t:f=w216:string)
                n104 = Bundle By Name(cluster=w213, "SelfRef"=w221) -> (w224:T8)
                n105 = call <vilib>:"Add State(s) to Queue__jki_lib_state_machine.vi"("State(s) in Front (\"\")"="UI: Update Status >> DAQ Public Events.getDeviceIDN" ("State(s) in Front (\"\")"), "State(s) at Back (\"\")"=w216) -> ("States Out"=w214:string)  [unwired: 13 in]
                n106 = call <vilib>:"Add State(s) to Queue__jki_lib_state_machine.vi"("State(s) in Front (\"\")"=w214, "State(s) in (\"\")"=w226) -> ("States Out"=w225:string)  [unwired: 13 in]
              }
              event User Event {
                n107 = event-data() -> ("Calibration"=w232:T31)  [unwired: 1 in, 4 out]
                n108 = Unbundle By Name(w233) -> ("logConfiguration"=w230:bool)
                n109 = call "Is Value Changed.vim"("value"=w232) -> ("changed or first call?"=w231:bool)
                n110 = Unbundle By Name(w233) -> ("SelfRef"=w239:refnum<class "Instrument.Lockin.lvclass">)
                n111 = Bundle By Name(cluster=w239, "Calibration"=w232) -> (w237:refnum<class "Instrument.Lockin.lvclass">)
                n112 = And(x=w231, y=w230) -> (x .and. y?=w229:bool)
                n113 = Select(t="UI: Update Status >> Log: Log Configuration\nLog: Log Configuration >> Devices" ("State(s) in Front (\"\")"), s=w229, f="") -> (s? t:f=w235:string)
                n114 = Bundle By Name(cluster=w233, "SelfRef"=w237) -> (w240:T8)
                n115 = call <vilib>:"Add State(s) to Queue__jki_lib_state_machine.vi"("State(s) in Front (\"\")"="UI: Update Status >> DAQ Public Events.getCalibration" ("State(s) in Front (\"\")"), "State(s) at Back (\"\")"=w235) -> ("States Out"=w234:string)  [unwired: 13 in]
                n116 = call <vilib>:"Add State(s) to Queue__jki_lib_state_machine.vi"("State(s) in Front (\"\")"=w234, "State(s) in (\"\")"=w242) -> ("States Out"=w241:string)  [unwired: 13 in]
              }
              event User Event {
                n117 = event-data() -> ("Interval"=w243:u32)  [unwired: 1 in]
                n118 = Equal To 0?(x=w243) -> (x = 0?=w247:bool)
                n119 = Select(t=Lockin.Logging_Mode--Enum."disabled" ("Logging.Mode"), s=w247, f=Lockin.Logging_Mode--Enum."enabled" ("Logging.Mode")) -> (s? t:f=w244:T2)
                n120 = Unbundle By Name(w254) -> ("SelfRef"=w251:refnum<class "Instrument.Lockin.lvclass">)
                n121 = case shown="\"enabled\", Default" w244 {
                  tunnel: ["Open" ("input 1") "Close" ("input 1")] -> w248
                  frame "enabled", Default {
                  }
                  frame "disabled" {
                  }
                }
                n122 = Bundle By Name(cluster=w251, "Loggin mode"=w244, "Logging interval (ms)"=w243) -> (w253:refnum<class "Instrument.Lockin.lvclass">)
                n123 = Format Into String(format string="UI: Update Status >> Lockin Private Events.setLogMode\nUI: Front Panel State >> %s" ("State(s) in Front (\"\")"), w248) -> (resulting string=w249:string)  [unwired: 2 in, 1 out]
                n124 = Bundle By Name(cluster=w254, "SelfRef"=w253) -> (w255:T8)
                n125 = call <vilib>:"Add State(s) to Queue__jki_lib_state_machine.vi"("State(s) in Front (\"\")"=w249, "State(s) in (\"\")"=w257) -> ("States Out"=w256:string)  [unwired: 13 in]
              }
              event User Event {
                n126 = event-data() -> ("logConfiguration"=w260:bool)  [unwired: 1 in]
                n127 = Unbundle By Name(w264) -> ("SelfRef"=w262:refnum<class "Instrument.Lockin.lvclass">)
                n128 = Bundle By Name(cluster=w264, "SelfRef"=w262, "logConfiguration"=w260) -> (w265:T8)
                n129 = call <vilib>:"Add State(s) to Queue__jki_lib_state_machine.vi"("State(s) in Front (\"\")"="UI: Update Status >> Lockin Private Events.LogConfiguration\nUI: Update Status >> Log: Log Configuration\nLog: Log Configuration >> System\nLog: Log Configuration >> Devices\nLog: Log Configuration >> AO\nLog: Log Configuration >> AI\nLog: Log Configuration >> MCLI" ("State(s) in Front (\"\")"), "State(s) in (\"\")"=w267) -> ("States Out"=w266:string)  [unwired: 13 in]
              }
            }
          }
          frame "---------- Core ----------" {
            # "Do not put any code in this frame.\n(it is a separator no-op)"
            n130 = call <vilib>:"Add State(s) to Queue__jki_lib_state_machine.vi"("State(s) in (\"\")"=w272) -> ("States Out"=w271:string)  [unwired: 14 in]
          }
          frame Default {
            w283 = 42 items=["No error", "Argument error", "Memory is full", "Out of zone", "End of file", "File already open", "Generic file I/O error", "File not found", "File permission error", "Disk is full", "Duplicate path", "Too many files open", "System feature not enabled", "Resource file not found", "Cannot add resource", "Resource not found", "Image not found", "Image memory error", "Pen does not exist", "Config type invalid", "Config token not found", "Config parse error", "Config memory error", "Bad external code format", "Bad external code offset", "External code not present", "Null window", "Destroy window error", "Null menu", "Print aborted", "Bad print record", "Print driver error", "Windows error during printing", "Memory error during printing", "Print dialog error", "Generic print error", "Invalid device refnum", "Device not found", "Device parameter error", "Device unit error", "Cannot open device", "Device call aborted", "Generic error", "Cancelled by user", "Object ID too low", "Object ID too high", "Object not in heap", "Unknown heap", "Unknown object (invalid DefProc)", "Unknown object (DefProc not in table)", "Message out of range", "Invalid (null) method", "Unknown message", "Manager call not supported", "Bad address", "Network operation in progress", "Network operation timed out", "Connection is busy", "Network attribute not supported", "Network error", "Address in use", "System out of memory", "Connection aborted", "Connection refused", "Not connected", "Already connected", "Connection closed", "Initialization error (interapplication manager)", "Bad occurrence", "Wait on unbound occurrence handler", "Occurrence queue overflow", "Datalog type conflict", "Unused", "Unrecognized type (interapplication manager)", "Memory corrupt", "Failed to make temporary DLL", "Old CIN version", "Drag socket not found", "Failed to load drop-object", "Failed to register OLE object", "Failed to release OLE object", "Format specifier type mismatch", "Unknown format specifier", "Too few format specifiers", "Too many format specifiers", "Scan failed", "Newer CIN version", "Error converting to variant", "Runtime menu error", "Password tampered", "Variant attribute not found", "Incompatible variant data type", "Event data is not available", "Event Store is not present", "Occurrence is not found", "Event Queue is not created", "Event info is not available", "Refnum passed is NULL", "Error retrieving Class GUID", "Error retrieving CoClass GUID", "Error retrieving TypeLib GUID.", "Bad built application magic bytes.", "Specific driver is different from the specific driver associated with the Logical Name.", "There is no session opened to the class driver.", "Max Error", "MAX - Error with config objects", "MAX - Error loading configuration", "MAX - Group not supported"]
            # "Current State"
            # "Do not delete, rename, or modify this frame.\n(this is used to capture unhandled states and typos)"
            # "Handle mistyped state name (developer tool)"
            n131 = Format Into String(format string="Software Exception: Unhandled State \"%s\"." ("message"), error in=w279, w274) -> (resulting string=w282:string, error out=w281:errorcluster)  [unwired: 1 in]
            n132 = call <vilib>:"Error Cluster From Error Code.vi"("show call chain? (False)"=TRUE, "error in (no error)"=w281, "error message (\"\")"=w282, "error code (0)"=w283) -> ("error out"=w280:errorcluster)  [unwired: 5 in]
            n133 = call <vilib>:"Add State(s) to Queue__jki_lib_state_machine.vi"("State(s) in (\"\")"=w278) -> ("States Out"=w277:string)  [unwired: 14 in]
          }
          frame "Initialize Core Data" {
            # "Do not delete, rename, or modify this frame.\n(this is used to determine panel behavior on exit)"
            # "originally closed?"
            # "exe?"
            # "If panel starts closed or is an EXE, then close it when we exit"
            n134 = property class="VI"() -> ("Front Panel.Open"=w293:bool)  [unwired: 2 in, 2 out]
            n135 = property class="App"() -> ("App.Kind"=w292:T3)  [unwired: 2 in, 2 out]
            n136 = control-ref of="Current VI Reference"() -> (w286:refnum<vi>)
            n137 = Not(x=w293) -> (.not. x?=w290:bool)
            n138 = Equal?(x=w292, y=T3."Run Time System" ("Application:Kind")) -> (x = y?=w289:bool)
            n139 = Or(x=w290, y=w289) -> (x .or. y?=w287:bool)
            n140 = Bundle By Name(cluster=w288, "Core.Current VI Reference"=w286, "Core.Close Panel on Exit?"=w287) -> (w295:T8)
            n141 = call <vilib>:"Add State(s) to Queue__jki_lib_state_machine.vi"("State(s) in (\"\")"=w297) -> ("States Out"=w296:string)  [unwired: 14 in]
          }
          frame "Error Handler" {
            w300 = FALSE  # Stop on Unhandled Error (T)
            # "Clear error"
            # "There was an error while handling the error.\nStop the process. This error can only occur if public events references are invalid or if the state machine object is destroyed."
            # "Overwrite this method to handle errors and pass to parent if not handled. Parent will fire a public event if the error is not handled up the chain of classes."
            n142 = Unbundle By Name(w306) -> ("SelfRef"=w309:refnum<class "Instrument.Lockin.lvclass">)
            n143 = call-dynamic "Handle Error.vi"("Stop on Unhandled Error (T)"=w300, "error in"=w308, "SMO"=w309) -> ("handling error"=w301:errorcluster, "Unhandled error"=w303:errorcluster)  [unwired: 6 in, 1 out]
            n144 = Bundle By Name(cluster=w306, "Core.Last Error.remaining states"=w299, "Core.Last Error.error"=w303) -> (w305:T8)
            n145 = Select(t="Exit", s=w301, f="Macro: Post Error Handling") -> (s? t:f=w304:string)
          }
          frame "Exit" {
            # "Do not put any code in this frame.\n(No errors that occur here will be handled.)"
            n146 = Unbundle By Name(w312) -> ("Core.Last Error.error"=w311:errorcluster)
            n147 = call <vilib>:"Add State(s) to Queue__jki_lib_state_machine.vi"("State(s) in (\"\")"=w316) -> ("States Out"=w315:string)  [unwired: 14 in]
          }
          frame "---------- Data ----------" {
            # "Do not put any code in this frame.\n(It is a separator no-op. You can make a copy of this frame to create a new Data frame)"
            n148 = call <vilib>:"Add State(s) to Queue__jki_lib_state_machine.vi"("State(s) in (\"\")"=w321) -> ("States Out"=w320:string)  [unwired: 14 in]
          }
          frame "Data: Initialize" {
            w322 = FALSE  # logConfiguration
            w323 = T6 {"AO"=[], "AI"=[], "X"=[], "Y"=[]}  # SweepWaveformsBuffer
            w328 = T33 {"Current VI Reference"=refnum, "Close Panel on Exit?"=FALSE, "Last Error"={"error"={"status"=FALSE, "code"=0, "source"=""}, "previous state"="", "remaining states"=""}, "Shutdown?"=FALSE}  # Core
            # "do not delete - used by framework"
            # "Data names and types of shift register data are defined by this bundle."
            # "Initialize the shift-register data, here.\n(data names are defined by what you wire into the bundle function)"
            n149 = Bundle By Name(cluster=w326, "Loggin mode"=Lockin.Logging_Mode--Enum."disabled" ("Mode"), "Logging interval (ms)"=u32 1000 ("Logging.Interval (s)")) -> (w327:refnum<class "Instrument.Lockin.lvclass">)
            n150 = Bundle("Core"=w328, "SelfRef"=w327, "logConfiguration"=w322, "SweepWaveformsBuffer"=w323) -> (w331:T8)  [unwired: 1 in]
            n151 = call <vilib>:"Add State(s) to Queue__jki_lib_state_machine.vi"("State(s) in (\"\")"=w333) -> ("States Out"=w332:string)  [unwired: 14 in]
          }
          frame "Data: Cleanup" {
            # "Cleanup any data and references, here.\n(this is called automatically, by the Macro: Exit)"
            n152 = Unbundle By Name(w335) -> ("Core.Current VI Reference"=w338:refnum<vi>)
            n153 = Close Reference(reference=w338, error in (no error)=w337) -> (error out=w336:errorcluster)
            n154 = call <vilib>:"Add State(s) to Queue__jki_lib_state_machine.vi"("State(s) in (\"\")"=w340) -> ("States Out"=w339:string)  [unwired: 14 in]
          }
          frame "Data: Buffer" {
            # "Data: Buffer\n()"
            n155 = Unbundle By Name(w349) -> ("SweepWaveformsBuffer.AO"=w346:waveform(dbl)[], "SweepWaveformsBuffer.AI"=w345:waveform(dbl)[], "SweepWaveformsBuffer.X"=w343:waveform(dbl)[], "SweepWaveformsBuffer.Y"=w344:waveform(dbl)[], "SelfRef"=w341:refnum<class "Instrument.Lockin.lvclass">)
            n156 = Unbundle By Name(w341) -> ("AO"=w355:waveform(dbl)[], "AI"=w354:waveform(dbl)[], "X"=w353:waveform(dbl)[], "Y"=w352:waveform(dbl)[])
            n157 = call "Waveform Buffer.vi"("Waveform B []"=w355, "Waveforrm A []"=w346) -> ("Waveform out []"=w348:waveform(dbl)[])  [unwired: 8 in, 1 out]
            n158 = call "Waveform Buffer.vi"("Waveform B []"=w354, "Waveforrm A []"=w345) -> ("Waveform out []"=w342:waveform(dbl)[])  [unwired: 8 in, 1 out]
            n159 = call "Waveform Buffer.vi"("Waveform B []"=w353, "Waveforrm A []"=w343) -> ("Waveform out []"=w347:waveform(dbl)[])  [unwired: 8 in, 1 out]
            n160 = call "Waveform Buffer.vi"("Waveform B []"=w352, "Waveforrm A []"=w344) -> ("Waveform out []"=w351:waveform(dbl)[])  [unwired: 8 in, 1 out]
            n161 = Bundle By Name(cluster=w349, "SweepWaveformsBuffer.AO"=w348, "SweepWaveformsBuffer.AI"=w342, "SweepWaveformsBuffer.X"=w347, "SweepWaveformsBuffer.Y"=w351) -> (w350:T8)
            n162 = call <vilib>:"Add State(s) to Queue__jki_lib_state_machine.vi"("State(s) in (\"\")"=w359) -> ("States Out"=w358:string)  [unwired: 14 in]
          }
          frame "---------- UI ----------" {
            # "Do not put any code in this frame.\n(It is a separator no-op. You can make a copy of this frame to create a new UI frame)"
            n163 = call <vilib>:"Add State(s) to Queue__jki_lib_state_machine.vi"("State(s) in (\"\")"=w364) -> ("States Out"=w363:string)  [unwired: 14 in]
          }
          frame "UI: Initialize" {
            # "Initialize the User Interface, here.\n(this is called automatically, by the Macro: Init)"
            n164 = call <userlib>:"Fit VI window to Largest Dec__ogtk.vi"("error in (no error)"=w366, "border spacing (2 px)"=0) -> ("error out"=w367:errorcluster)  [unwired: 4 in, 1 out]
            n165 = call <vilib>:"Add State(s) to Queue__jki_lib_state_machine.vi"("State(s) in (\"\")"=w372) -> ("States Out"=w371:string)  [unwired: 14 in]
            "String" <- "" ("String")
          }
          frame "UI: Update Status" {
            n166 = call <userlib>:"State History.vi"("Current State"=w373) -> ("History"=w374:string)  [unwired: 9 in, 1 out]
            n167 = local write "String"(w374) -> ()
            n168 = call <vilib>:"Add State(s) to Queue__jki_lib_state_machine.vi"("State(s) in (\"\")"=w379) -> ("States Out"=w378:string)  [unwired: 14 in]
          }
          frame "UI: Wait" {
            # "Do not put any code in this frame.\n(It is a separator no-op. You can make a copy of this frame to create a new UI frame)"
            n169 = Scan From String(format string="%d", input string=w380, default 1=u32 0 ("default value 1")) -> (output 1=w381:u32)  [unwired: 2 in, 3 out]
            n170 = Wait (ms)(milliseconds to wait=w381) -> ()  [unwired: 1 out]
            n171 = call <vilib>:"Add State(s) to Queue__jki_lib_state_machine.vi"("State(s) in (\"\")"=w388) -> ("States Out"=w387:string)  [unwired: 14 in]
          }
          frame "UI: Cursor Set" {
            # "Argument"
            # "Initialize the User Interface, here.\n(this is called automatically, by the Macro: Init)"
            n172 = disable-structure shown="Default" {
              disable-tunnel: w391 -> [w396 w399]
              disable-tunnel: [w396 w398] -> w390
              disable-tunnel: w389 -> [_ w397]
              frame condition #0 {
              }
              frame condition #1 (active) {
                n173 = case shown="\"Idle\", Default" w397 {
                  tunnel: w399 -> [w401 w403]
                  tunnel: [w400 w402] -> w398
                  frame "Idle", Default {
                    n174 = call <vilib>:"Unset Busy.vi"("error in (no error)"=w401) -> ("error out"=w400:errorcluster)  [unwired: 10 in]
                  }
                  frame "Busy" {
                    n175 = call <vilib>:"Set Busy.vi"("error in (no error)"=w403) -> ("error out"=w402:errorcluster)  [unwired: 9 in, 1 out]
                  }
                }
              }
            }
            n176 = call <vilib>:"Add State(s) to Queue__jki_lib_state_machine.vi"("State(s) in (\"\")"=w395) -> ("States Out"=w394:string)  [unwired: 14 in]
          }
          frame "UI: Front Panel State" {
            # "Argument"
            # "Set Front Panel Open or Closed\n(Usage: \"UI: Front Panel State >> Open|Close\")"
            n177 = Unbundle By Name(w407) -> ("Core.Current VI Reference"=w406:refnum<vi>)
            n178 = disable-structure shown="Default" {
              disable-tunnel: w409 -> [w415 w438]
              disable-tunnel: [w414 w438] -> w408
              disable-tunnel: w406 -> [w413 _]
              disable-tunnel: w405 -> [w412 _]
              frame condition #0 (active) {
                n179 = case shown="\"Close\"" w412 {
                  tunnel: w415 -> [w419 w432]
                  tunnel: [w421 w433] -> w414
                  tunnel: w413 -> [w420 w430]
                  frame "Open", Default {
                    n180 = property class="VI"(reference=w420, error in=w419) -> (reference out=w417:refnum<vi>, error out=w418:errorcluster, "FP.State"=w416:T4)
                    n181 = case shown="\"Closed\"" w416 {
                      tunnel: [w424 w427] -> w421
                      tunnel: w418 -> [w423 w427]
                      tunnel: w417 -> [w422 _]
                      frame "Closed" {
                        n182 = invoke class="VI" method="FP.Open"(reference=w422, error in=w423, "Activate"=TRUE, "State"=T4."Standard") -> (error out=w424:errorcluster)  [unwired: 1 in, 4 out]
                      }
                      frame Default {
                      }
                    }
                  }
                  frame "Close" {
                    n183 = property class="VI"(reference=w430, error in=w432) -> (reference out=w429:refnum<vi>, error out=w431:errorcluster, "FP.State"=w428:T4)
                    n184 = case shown="Default" w428 {
                      tunnel: [w434 w437] -> w433
                      tunnel: w431 -> [w434 w436]
                      tunnel: w429 -> [_ w435]
                      frame "Invalid", "Closed" {
                      }
                      frame Default {
                        n185 = invoke class="VI" method="FP.Close"(reference=w435, error in=w436) -> (error out=w437:errorcluster)  [unwired: 1 in, 2 out]
                      }
                    }
                  }
                }
              }
              frame condition #1 {
              }
            }
            n186 = call <vilib>:"Add State(s) to Queue__jki_lib_state_machine.vi"("State(s) in (\"\")"=w411) -> ("States Out"=w410:string)  [unwired: 14 in]
          }
          frame "---------- Macro ----------" {
            # "Do not put any code in this frame.\n(It is a separator no-op. You can make a copy of this frame to create a new Macro frame)"
            n187 = call <vilib>:"Add State(s) to Queue__jki_lib_state_machine.vi"("State(s) in (\"\")"=w443) -> ("States Out"=w442:string)  [unwired: 14 in]
          }
          frame "Macro: Initialize" {
            w445 = "UI: Initialize\nUI: Front Panel State >> Close\nMacro: Debug"  # UI: Initialize UI: Front Panel State >> Close Macro: Debug
            # "Initialization Macro\n(This is called once, when the VI starts)"
            n188 = call <vilib>:"Add State(s) to Queue__jki_lib_state_machine.vi"("State(s) in Front (\"\")"="Data: Initialize\nInitialize Core Data\nEvents: Register", "State(s) in (\"\")"="Process: Sync", "State(s) at Back (\"\")"=w445) -> ("States Out"=w448:string)  [unwired: 12 in]
            n189 = call <vilib>:"Add State(s) to Queue__jki_lib_state_machine.vi"("State(s) in Front (\"\")"=w448, "State(s) in (\"\")"=w452) -> ("States Out"=w451:string)  [unwired: 13 in]
          }
          frame "Macro: Post Error Handling" {
            # "Clear Last Error?"
            n190 = Unbundle By Name(w453) -> ("Core.Last Error.remaining states"=w456:string, "Core.Shutdown?"=w457:bool)
            n191 = Unbundle By Name(w453) -> ("Core.Last Error.error"=w460:errorcluster)
            n192 = case shown="False" FALSE {
              tunnel: w460 -> [w468 _]
              tunnel: [w468 _] -> w459
              frame False {
              }
              frame True {
              }
            }
            n193 = case shown="False" w457 {
              tunnel: w456 -> [w465 w467]
              tunnel: [w465 w466] -> w455
              frame False {
                # "These are the remaining states (at the moment the error occured). States can be altered according to business logic."
                # "NOT SHUTTING DOWN"
              }
              frame True {
                # "Developer can decide to alter the states but should be aware that during the shutdown process, there are certain states that must be run for the SMO to properly shut itself (and this process) down. As such, one can add states to perform additional clean-ups, but should append the remaining state to be executed."
                # "SHUTTING DOWN"
                n194 = call <vilib>:"Add State(s) to Queue__jki_lib_state_machine.vi"("State(s) in (\"\")"=w467) -> ("States Out"=w466:string)  [unwired: 14 in]
              }
            }
            n195 = Bundle By Name(cluster=w453, "Core.Last Error.error"=w459) -> (w454:T8)
            n196 = call <vilib>:"Add State(s) to Queue__jki_lib_state_machine.vi"("State(s) in Front (\"\")"=w455, "State(s) in (\"\")"=w464) -> ("States Out"=w463:string)  [unwired: 13 in]
          }
          frame "Macro: Debug" {
            # "exe?"
            # "If pane is an EXE, then close it when we exit"
            # "Macro: Debug\n(get debug behavior, determine UI and determine shutdown behavior)"
            n197 = Unbundle By Name(w472) -> ("Core.Close Panel on Exit?"=w475:bool, "SelfRef"=w480:refnum<class "Instrument.Lockin.lvclass">)
            n198 = property class="App"() -> ("App.Kind"=w478:T3)  [unwired: 2 in, 2 out]
            n199 = Equal?(x=w478, y=T3."Run Time System" ("Application:Kind")) -> (x = y?=w474:bool)
            n200 = call <userlib>:"Get Debug Mode.vi"("error in (no error)"=w469, "SMO"=w480) -> ("error out"=w470:errorcluster, "Behavior"=w479:T34)  [unwired: 7 in, 1 out]
            n201 = case shown="\"Normal\", Default" w479 {
              tunnel: [w484 w486] -> w476
              tunnel: w475 -> [w484 _]
              tunnel: w474 -> [_ w488]
              tunnel: [_ "UI: Front Panel State >> Open\nUI: Wait >> 1000"] -> w471
              frame "Normal", Default {
                # "respect core.close"
              }
              frame "Debug" {
                # "keep panel open\nunless exe"
                n202 = Or(x=w488, y=FALSE) -> (x .or. y?=w486:bool)
              }
            }
            n203 = Bundle By Name(cluster=w472, "Core.Close Panel on Exit?"=w476) -> (w473:T8)
            n204 = call <vilib>:"Add State(s) to Queue__jki_lib_state_machine.vi"("State(s) in Front (\"\")"=w471, "State(s) in (\"\")"=w483) -> ("States Out"=w482:string)  [unwired: 13 in]
          }
          frame "Macro: Exit" {
            # "Exit Macro\n(This is called once, when the VI exits)"
            n205 = Unbundle By Name(w489) -> ("Core.Close Panel on Exit?"=w501:bool)
            n206 = Bundle By Name(cluster=w489, "Core.Shutdown?"=TRUE) -> (w490:T8)
            n207 = Select(t="UI: Front Panel State >> Close", s=w501, f="") -> (s? t:f=w498:string)
            n208 = call <vilib>:"Add State(s) to Queue__jki_lib_state_machine.vi"("State(s) in Front (\"\")"="Data: Cleanup\nEvents: Unregister", "State(s) in (\"\")"="Process: Sync", "State(s) at Back (\"\")"="Exit") -> ("States Out"=w493:string)  [unwired: 12 in]
            n209 = call <vilib>:"Add State(s) to Queue__jki_lib_state_machine.vi"("State(s) in (\"\")"=w498, "State(s) at Back (\"\")"=w493) -> ("States Out"=w497:string)  [unwired: 13 in]
            n210 = call <vilib>:"Add State(s) to Queue__jki_lib_state_machine.vi"("State(s) in Front (\"\")"=w497, "State(s) in (\"\")"=w504) -> ("States Out"=w503:string)  [unwired: 13 in]
          }
          frame "---------- Process ----------" {
            # "Template Separator\n(You can make a copy of, or modify, this frame)"
            n211 = call <vilib>:"Add State(s) to Queue__jki_lib_state_machine.vi"("State(s) in (\"\")"=w509) -> ("States Out"=w508:string)  [unwired: 14 in]
          }
          frame "Process: Sync" {
            n212 = Unbundle By Name(w517) -> ("SelfRef"=w513:refnum<class "Instrument.Lockin.lvclass">)
            n213 = call <vilib>:"WaitOnProcessSync.vi"("error in (no error)"=w512, "SMO"=w513) -> ("error out"=w511:errorcluster, "Don't run?"=w516:bool)  [unwired: 7 in, 1 out]
            n214 = Select(t="Data: Cleanup\nEvents: Unregister\nExit", s=w516, f="") -> (s? t:f=w510:string)
            n215 = call <vilib>:"Add State(s) to Queue__jki_lib_state_machine.vi"("State(s) in Front (\"\")"=w510, "State(s) in (\"\")"=w520) -> ("States Out"=w519:string)  [unwired: 13 in]
          }
          frame "---------- Events ----------" {
            # "Template Separator\n(You can make a copy of, or modify, this frame)"
            n216 = call <vilib>:"Add State(s) to Queue__jki_lib_state_machine.vi"("State(s) in (\"\")"=w525) -> ("States Out"=w524:string)  [unwired: 14 in]
          }
          frame "Events: Register" {
            # "Expand to add\nmore events"
            n217 = Unbundle By Name(w536) -> ("SelfRef"=w535:refnum<class "Instrument.Lockin.lvclass">)
            n218 = call <vilib>:"GetProtectedEvents.vi"("SMO"=w535) -> ("error out"=w537:errorcluster, "SMO Protected Events"=w539:T35, "SMO out"=w530:refnum<class "Instrument.Lockin.lvclass">)  [unwired: 8 in]
            n219 = call "Lockin.getDAQPublicEvents.vi"("Instrument.Lockin in"=w530) -> ("error out"=w531:errorcluster, "DAQ SMO Public Events"=w529:T36, "DAQ Public Events"=w532:T37, "Instrument.Lockin out"=w528:refnum<class "Instrument.Lockin.lvclass">)  [unwired: 7 in]
            n220 = call "Lockin.GetPrivateEvents.vi"("Instrument.Lockin in"=w528) -> ("error out"=w526:errorcluster, "Lockin Private Events"=w527:T38)  [unwired: 8 in, 1 out]
            n221 = register-events(w539, w532, w529, w527) -> (reference out=w540:refnum<event-registration>, error out=w533:errorcluster)  [unwired: 2 in]
            n222 = Merge Errors(w533, w526, w531, w537, w534) -> (w538:errorcluster)
            n223 = call <vilib>:"Add State(s) to Queue__jki_lib_state_machine.vi"("State(s) in (\"\")"=w542) -> ("States Out"=w541:string)  [unwired: 14 in]
          }
          frame "Events: Unregister" {
            n224 = Unregister For Events(event registration refnum=w545, error in=w544) -> (error out=w543:errorcluster)
            n225 = call <vilib>:"Clear Errors.vi"("error in (no error)"=w543) -> ()  [unwired: 5 in, 2 out]
            n226 = call <vilib>:"Add State(s) to Queue__jki_lib_state_machine.vi"("State(s) in (\"\")"=w548) -> ("States Out"=w547:string)  [unwired: 14 in]
          }
          frame "---------- Log ----------" {
            n227 = call <vilib>:"Add State(s) to Queue__jki_lib_state_machine.vi"("State(s) in (\"\")"=w553) -> ("States Out"=w552:string)  [unwired: 14 in]
          }
          frame "Log: Manager" {
            n228 = Unbundle By Name(w560) -> ("SelfRef"=w559:refnum<class "Instrument.Lockin.lvclass">)
            n229 = Unbundle By Name(w559) -> ("Logging interval (ms)"=w557:u32, "DAQ State"=w556:T5, "Loggin mode"=w555:T2)
            n230 = case shown="\"Sweep\"" w554 {
              selector: w554 -> [_ _ w582]
              tunnel: ["" ("State(s) in Front (\"\")") w571 w586] -> w558
              tunnel: w557 -> [_ _ w580]
              tunnel: w556 -> [_ w570 w585]
              tunnel: w555 -> [_ _ w584]
              frame Default {
              }
              frame "Sweep" {
                w566 = "UI: Update Status >> Log Sweep\nLog: Log Sweep" ("State(s) in Front (\"\")")
                n231 = Equal?(x=w570, y=Status--enum."sweeping") -> (x = y?=w574:bool)
                n232 = call <userlib>:"Periodic Trigger__ogtk.vi"("time (ms)"=u32 1000) -> ("Triggered"=w575:bool)  [unwired: 12 in, 2 out]
                n233 = Select(t="UI: Update Status >> Buffer Sweep\nData: Buffer" ("State(s) in Front (\"\")"), s=w574, f=w566) -> (s? t:f=w568:string)
                n234 = Select(t=w566, s=w575, f="") -> (s? t:f=w576:string)
                n235 = call <vilib>:"Add State(s) to Queue__jki_lib_state_machine.vi"("State(s) in Front (\"\")"=w568, "State(s) at Back (\"\")"=w576) -> ("States Out"=w571:string)  [unwired: 13 in]
              }
              frame "AO AI", "Results" {
                n236 = case shown="\"AO AI\"" w582 {
                  tunnel: ["UI: Update Status >> Log Results\nLog: Log Results" ("State(s) in Front (\"\")") "UI: Update Status >> Log AO\nLog: Log AO\nUI: Update Status >> Log AI\nLog: Log AI" ("State(s) in Front (\"\")")] -> w581
                  frame "Results", Default {
                  }
                  frame "AO AI" {
                  }
                }
                n237 = Not Equal?(x=w585, y=Status--enum."sweeping") -> (x != y?=w587:bool)
                n238 = Equal?(x=w584, y=Lockin.Logging_Mode--Enum."enabled") -> (x = y?=w577:bool)
                n239 = call <userlib>:"Periodic Trigger__ogtk.vi"("time (ms)"=w580) -> ("Triggered"=w578:bool)  [unwired: 12 in, 2 out]
                n240 = Compound Arithmetic op=AND(w578, w587, w577) -> (w579:bool)
                n241 = Select(t=w581, s=w579, f="" ("State(s) in Front (\"\")")) -> (s? t:f=w586:string)
              }
            }
            n242 = call <vilib>:"Add State(s) to Queue__jki_lib_state_machine.vi"("State(s) in Front (\"\")"=w558, "State(s) in (\"\")"=w564) -> ("States Out"=w563:string)  [unwired: 13 in]
          }
          frame "Log: Log Configuration" {
            n243 = Unbundle By Name(w598) -> ("SelfRef"=w597:refnum<class "Instrument.Lockin.lvclass">)
            n244 = Scan From String(input string=w592, default 1=enum16{"System", "Devices", "AO", "AI", "MCLI"}."AI" ("Enum")) -> (output 1=w593:enum16{"System", "Devices", "AO", "AI", "MCLI"})  [unwired: 3 in, 3 out]
            n245 = call "Log Configuration.vi"("error in (no error)"=w595, "Enum"=w593, "Instrument.Lockin in"=w597) -> ("error out"=w596:errorcluster)  [unwired: 7 in, 1 out]
            n246 = call <vilib>:"Add State(s) to Queue__jki_lib_state_machine.vi"("State(s) in (\"\")"=w601) -> ("States Out"=w600:string)  [unwired: 14 in]
          }
          frame "Log: Log AO" {
            n247 = Unbundle By Name(w605) -> ("SelfRef"=w602:refnum<class "Instrument.Lockin.lvclass">)
            n248 = call "Log AO.vi"("error in (no error)"=w603, "Instrument.Lockin in"=w602) -> ("error out"=w604:errorcluster)  [unwired: 8 in, 1 out]
            n249 = call <vilib>:"Add State(s) to Queue__jki_lib_state_machine.vi"("State(s) in (\"\")"=w608) -> ("States Out"=w607:string)  [unwired: 14 in]
          }
          frame "Log: Log AI" {
            n250 = Unbundle By Name(w612) -> ("SelfRef"=w610:refnum<class "Instrument.Lockin.lvclass">)
            n251 = call "Log AI.vi"("error in (no error)"=w609, "Instrument.Lockin in"=w610) -> ("error out"=w611:errorcluster)  [unwired: 8 in, 1 out]
            n252 = call <vilib>:"Add State(s) to Queue__jki_lib_state_machine.vi"("State(s) in (\"\")"=w615) -> ("States Out"=w614:string)  [unwired: 14 in]
          }
          frame "Log: Log Results" {
            n253 = Unbundle By Name(w619) -> ("SelfRef"=w618:refnum<class "Instrument.Lockin.lvclass">)
            n254 = call "Log Results.vi"("error in (no error)"=w617, "Instrument.Lockin in"=w618) -> ("error out"=w616:errorcluster)  [unwired: 8 in, 1 out]
            n255 = call <vilib>:"Add State(s) to Queue__jki_lib_state_machine.vi"("State(s) in (\"\")"=w622) -> ("States Out"=w621:string)  [unwired: 14 in]
          }
          frame "Log: Log Sweep" {
            w624 = waveform(dbl)[] [] ("AO_wfm")
            n256 = Unbundle By Name(w626) -> ("SelfRef"=w631:refnum<class "Instrument.Lockin.lvclass">, "SweepWaveformsBuffer"=w628:T6)
            n257 = call "Log Sweep.vi"("error in (no error)"=w630, "SweepWaveforms"=w628, "Instrument.Lockin in"=w631) -> ("error out"=w629:errorcluster)  [unwired: 8 in]
            n258 = Bundle By Name(cluster=T6 {"AO"=[], "AI"=[], "X"=[], "Y"=[]} ("SweepWaveformsBuffer"), "AO"=w624, "AI"=w624, "X"=w624, "Y"=w624) -> (w625:T6)
            n259 = Bundle By Name(cluster=w626, "SweepWaveformsBuffer"=w625) -> (w627:T8)
            n260 = call <vilib>:"Add State(s) to Queue__jki_lib_state_machine.vi"("State(s) in (\"\")"=w634) -> ("States Out"=w633:string)  [unwired: 14 in]
          }
        }
      }
    }
    frame Error {
    }
  }
  n261 = call-parent "Process.vi"("error in"=w5, "Instrument"=w4) -> ("error out"=w2:errorcluster, "Instrument out"=→"Instrument.Lockin out":refnum<class "Instrument.Lockin.lvclass">)  [unwired: 8 in]
  n262 = Merge Errors(w2, w1) -> (→"error out":errorcluster)
